vi "Periodic Tasks.vi"(8 "error in":errorcluster) -> ()   [LabVIEW 2015]
doc: "This VI runs in parallel to other tasks. It can contain as many user-defined periodic loops as you need. These can carry out PID or other sorts of timed response."
uses:
  <vilib>/Rock Robotics/WPI/Solenoid/WPI_SolenoidValue.ctl
  Robot Global Data.vi
  <vilib>/Rock Robotics/Network Tables/NT Write Boolean.vi
  <vilib>/Rock Robotics/WPI/Solenoid/WPI_SolenoidSetEnum.vi
  <vilib>/Rock Robotics/WPI/Utilities/WPI_GetSetVariantRefNum.vi
  <vilib>/Rock Robotics/WPI/RobotDrive/WPI_RobotDriveArcadeDrive_Standard(NoSaturation).vi
  <vilib>/Rock Robotics/Network Tables/NT Read Number.vi
  <vilib>/Rock Robotics/Network Tables/NT Read Numeric Array.vi
  <vilib>/Rock Robotics/Network Tables/NT Read Boolean.vi
  <vilib>/Rock Robotics/Network Tables/NT Write Number.vi
  navX Library v2/navX Library v2.lvlib
panel:
  in  "memoryStartAsSlow":dbl=0.3
  in  "min thresh 5":dbl=5e-05 format="%#_13g"
  in  "add if slow 5":dbl=0.007 format="%#_13g"
  in  "add if fast 5":dbl format="%#_13g"
  in  "turnSpeedStartSlow":dbl=0.3
  in  "distToStartAsSlow":dbl=0.2 format="%#_13g"
  in  "turnSpeedHard":dbl=0.5 format="%#_13g"
  in  "maxhi 2":dbl=0.8
  in  "high max 2":dbl=1.0
  in  "maxhi":dbl=0.65
  in  "turnSpeedSlow":dbl=0.37 format="%#_13g"
  in  "add if fast 4":dbl format="%#_13g"
  in  "add if slow 4":dbl=0.01 format="%#_13g"
  in  "min thresh 4":dbl=5e-05 format="%#_13g"
  out "aimState":i32
  in  "holding":dbl=0.25 format="%#_13g"
  in  "turnSpeed 7":dbl=0.37 format="%#_13g"
  in  "turnSpeedMedium":dbl=0.45 format="%#_13g"
  out "Target Angle 3":dbl=-17.534194944028258 format="%#_13g"
  in  "Angle 2":dbl=5.0 format="%#_13g"
  in  "cameraTarget 3":dbl=-0.03 format="%#_13g"
  in  "viewAngle 3":dbl=37.0 format="%#_13g"
  in  "arm vert offset":dbl=0.24 format="%#_13g"
  in  "arm horiz offset":dbl=0.07 format="%#_13g"
  out "leftOrRight":dbl=1.0
  in  "aimTolerance 2":dbl=6.0
  in  "high max":dbl=1.0
  in  "tapeRuntime":i32=25
  out "timeSaved 3":i32=27312
  in  "shiftthesh":dbl=0.67 format="%#_13g"
  in  "practiceOffset":dbl=-0.025 format="%#_13g"
  in  "tapeInPTO":dbl=-0.7
  out "timeSaved 2":i32=27123
  in  "left wait time":u32=13
  out "timeSaved":i32=14839
  in  "right wait time":u32=7
  out "LeftPin":bool
  out "RightPin":bool=TRUE
  in  "tapeOut":dbl=1.0 format="%#_13g"
  in  "tapeIn":dbl=-0.5 format="%#_13g"
  in  "tapeReturnSpeed":dbl
  in  "PTO speed":dbl=-1.0 format="%#_13g"
  in  "forceLowGear":bool
  out "voltage (V) 3":dbl=12.15
  out "Retainer Locked On":bool
  in  "y-override speed":dbl=-0.6 format="%#_13g"
  in  "Y-overide":bool
  in  "aimBot":dbl
  in  "modifyArm":dbl
  in  "distToRaise":dbl=24.0 format="%#_13g"
  in  "distToLower":dbl format="%#_13g"
  out "arm pot":dbl=0.9054580314226414
  out "rememberEnc":dbl=43.89548625
  out "Yes":bool
  in  "arm cdf offset":dbl=0.12
  in  "intake hi":dbl=-0.8
  out "arm output":dbl=-0.0 format="%.2f"
  # "This is all related to the auto-aim"
  # "These are what happens when starting close to the goal"
  # "ARM STUFF"
  # "auto-CDF"
  # "affects drive train:"
  # "minor high gear restrictions"
  # "Everything related to tape measures"
  # "9 and 16"
  # "practice 11 and 19"
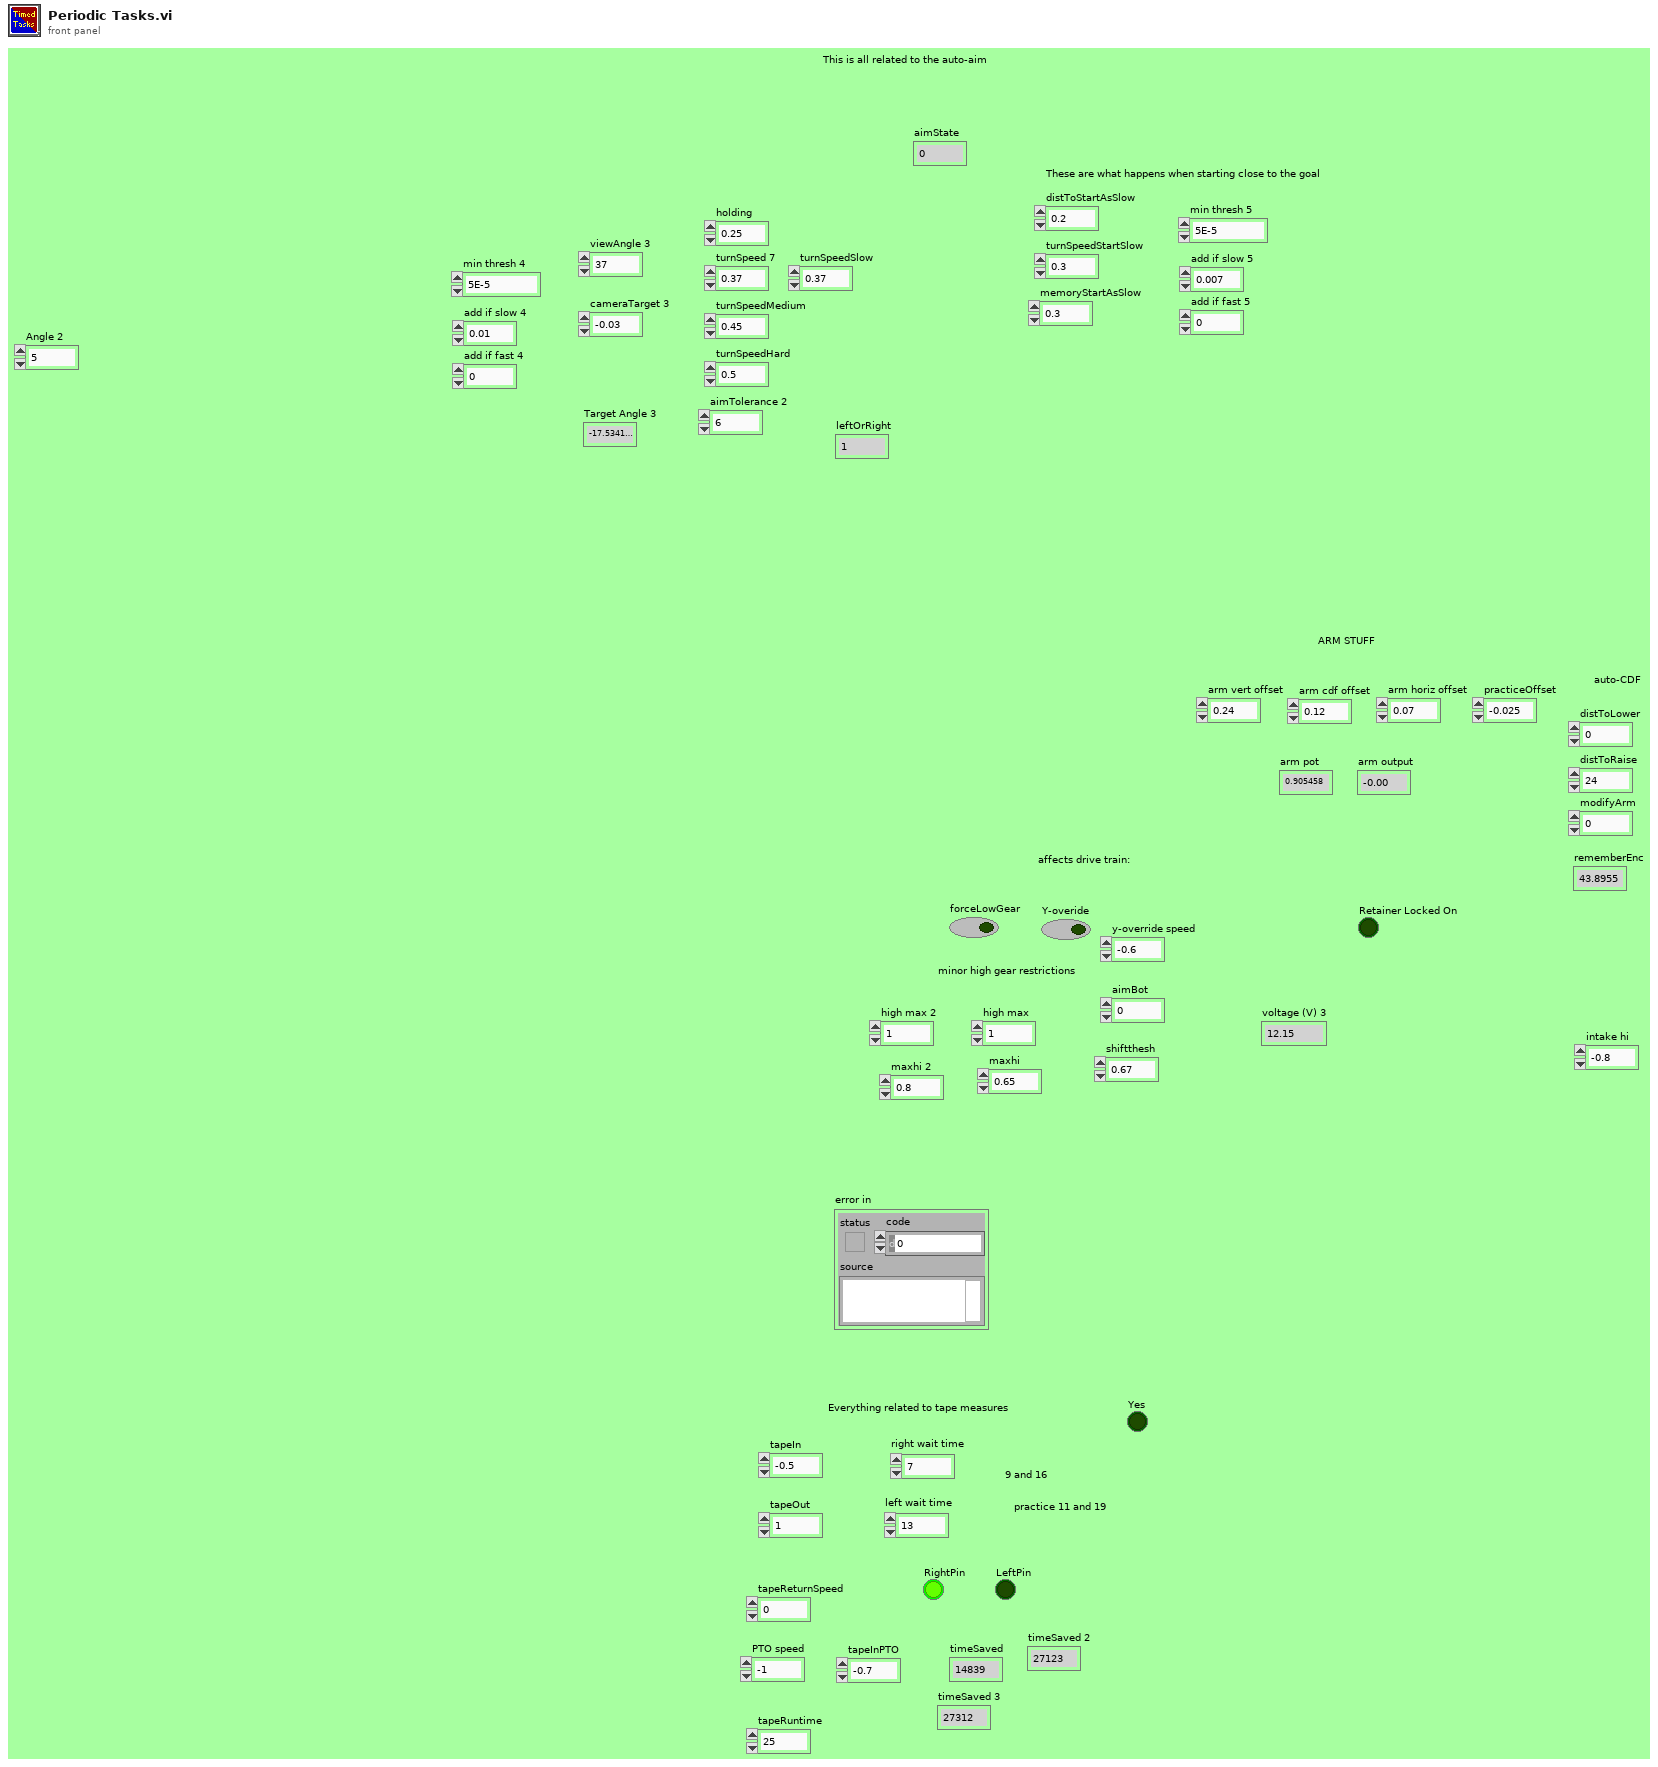
[diagram p1: front panel]
types:
  T1 = typedef "WPI_SolenoidDevRef.ctl" = cluster{"DevStatus":errorcluster, "Pneumatics Control Module":u8, "Forward Solenoid Channel":T2, "Reverse Solenoid Channel":T2}
  T2 = typedef "WPI_SolenoidChannel.ctl" = enum8{"Solenoid 0", "Solenoid 1", "Solenoid 2", "Solenoid 3", "Solenoid 4", "Solenoid 5", "Solenoid 6", "Solenoid 7", "Invalid"}
  T3 = typedef "WPI_RobotDriveDevRef.ctl" = cluster{"DevStatus":errorcluster, "Motors[]":T4[], "Square Inputs":bool, "Max Output":dbl}
  T4 = typedef "WPI_MotorControlDeviceRef.ctl" = cluster{"DeviceStatus":errorcluster, "Type":T5, "PWM":cluster{"PWM Channel":T6, "DeadBand":T7}, "CAN":cluster{"Device Number":u8, "Control Mode":T8, "Semaphore":T9, "Max Vout":dbl, "TalonSRX Control Mode":T10}, "Invert":bool}
  T5 = typedef "WPI_MotorControlType.ctl" = enum16{"PWM", "CAN", "CANTalonSRX"}
  T6 = typedef "FPGA_DIOPWMChannel.ctl" = enum8{"PWM 0", "PWM 1", "PWM 2", "PWM 3", "PWM 4", "PWM 5", "PWM 6", "PWM 7", "PWM 8", "PWM 9", "PWM MXP 0", "PWM MXP 1", "PWM MXP 2", "PWM MXP 3", "PWM MXP 4", "PWM MXP 5", "PWM MXP 6", "PWM MXP 7", "PWM MXP 8", "PWM MXP 9", "Invalid"}
  T7 = typedef "WPI_PWMDeadband.ctl" = cluster{"Name":string, "maxPositivePwm":i32, "minPositivePwm":i32, "centerPwm":i32, "maxNegativePwm":i32, "minNegativePwm":i32, "angularRange":u16}
  T8 = typedef "WPI_CANJaguar_ControlMode.ctl" = enum8{"Percent VBus", "Current", "Speed", "Position", "Voltage"}
  T9 = typedef "Semaphore RefNum" = refnum<k1>
  T10 = typedef "WPI_CANTalonSRX_APIControlMode.ctl" = enum8{"Percent VBus", "Speed", "Position", "Slave", "Unchanged / Invalid", "Voltage Compensation", "Current", "Motion Profile"}
  T11 = typedef "WPI_EncoderDevRef.ctl" = cluster{"DevStatus":errorcluster, "EncoderIndex":T12, "CounterIndex":T13, "DistancePerCount":dbl, "Decoding Type":T14}
  T12 = typedef "FPGA_EncoderIdx.ctl" = enum8{"Enc 0", "Enc 1", "Enc 2", "Enc 3", "Enc 4", "Enc 5", "Enc 6", "Enc 7", "Invalid"}
  T13 = typedef "FPGA_CounterCtrSystemIndex.ctl" = enum8{"Ctr 0", "Ctr 1", "Ctr 2", "Ctr 3", "Ctr 4", "Ctr 5", "Ctr 6", "Ctr 7", "Invalid"}
  T14 = typedef "WPI_EncoderType.ctl" = enum16{"1x", "2x", "4x"}
  T15 = typedef "WPI_DigitalInputDevRef.ctl" = cluster{"DevStatus":errorcluster, "DIO Channel":T16}
  T16 = typedef "FPGA_DIOChannel.ctl" = enum8{"DIO 0", "DIO 1", "DIO 2", "DIO 3", "DIO 4", "DIO 5", "DIO 6", "DIO 7", "DIO 8", "DIO 9", "DIO MXP 0", "DIO MXP 1", "DIO MXP 2", "DIO MXP 3", "DIO MXP 4", "DIO MXP 5", "DIO MXP 6", "DIO MXP 7", "DIO MXP 8", "DIO MXP 9", "DIO MXP 10", "DIO MXP 11", "DIO MXP 12", "DIO MXP 13", "DIO MXP 14", "DIO MXP 15", "Invalid"}
  T17 = typedef "WPI_PotentiometerDevRef.ctl" = cluster{"DevStatus":errorcluster, "Analog Channel":T18, "Invert Output":bool}
  T18 = typedef "FPGA_AIChannel.ctl" = enum8{"AI 0", "AI 1", "AI 2", "AI 3", "AI MXP 0", "AI MXP 1", "AI MXP 2", "AI MXP 3", "Invalid"}
  T19 = typedef "WPI_AnalogChannelDevRef.ctl" = cluster{"DevStatus":errorcluster, "Analog Channel":T18}
  T20 = typedef "navX Library v2.lvlib/Z900_navX_DeviceTypeDef.ctl" = cluster{"Interface":cluster{"Protocol":T21, "Update Rate (4Hz-60Hz)":u8, "navX Open TypeDef":variant}, "Notify Packet":refnum<notifier>, "Loop VI Refnum":refnum<vi>, "Ready to Close Occurrence Refnum":refnum<k4>}
  T21 = typedef "navX Library v2.lvlib/Z900_navX_ProtocolTypeDef.ctl" = enum16{"SERIAL", "I2C", "SPI"}
  T22 = typedef "WPI_CompressorDevRef.ctl" = cluster{"DevStatus":errorcluster, "Pneumatics Control Module":u8}
  T23 = cluster{"Yaw":dbl, "Roll":dbl, "Pitch":dbl, "Heading":dbl, "Fused Heading":dbl}
  T24 = typedef "WPI_SolenoidValue.ctl" = enum16{"Off", "On", "Forward", "Reverse"}
  T25 = cluster{"SolenoidDevRef":T1, "SolenoidDevRef":T1, "SolenoidDevRef":T1, "SolenoidDevRef":T1}
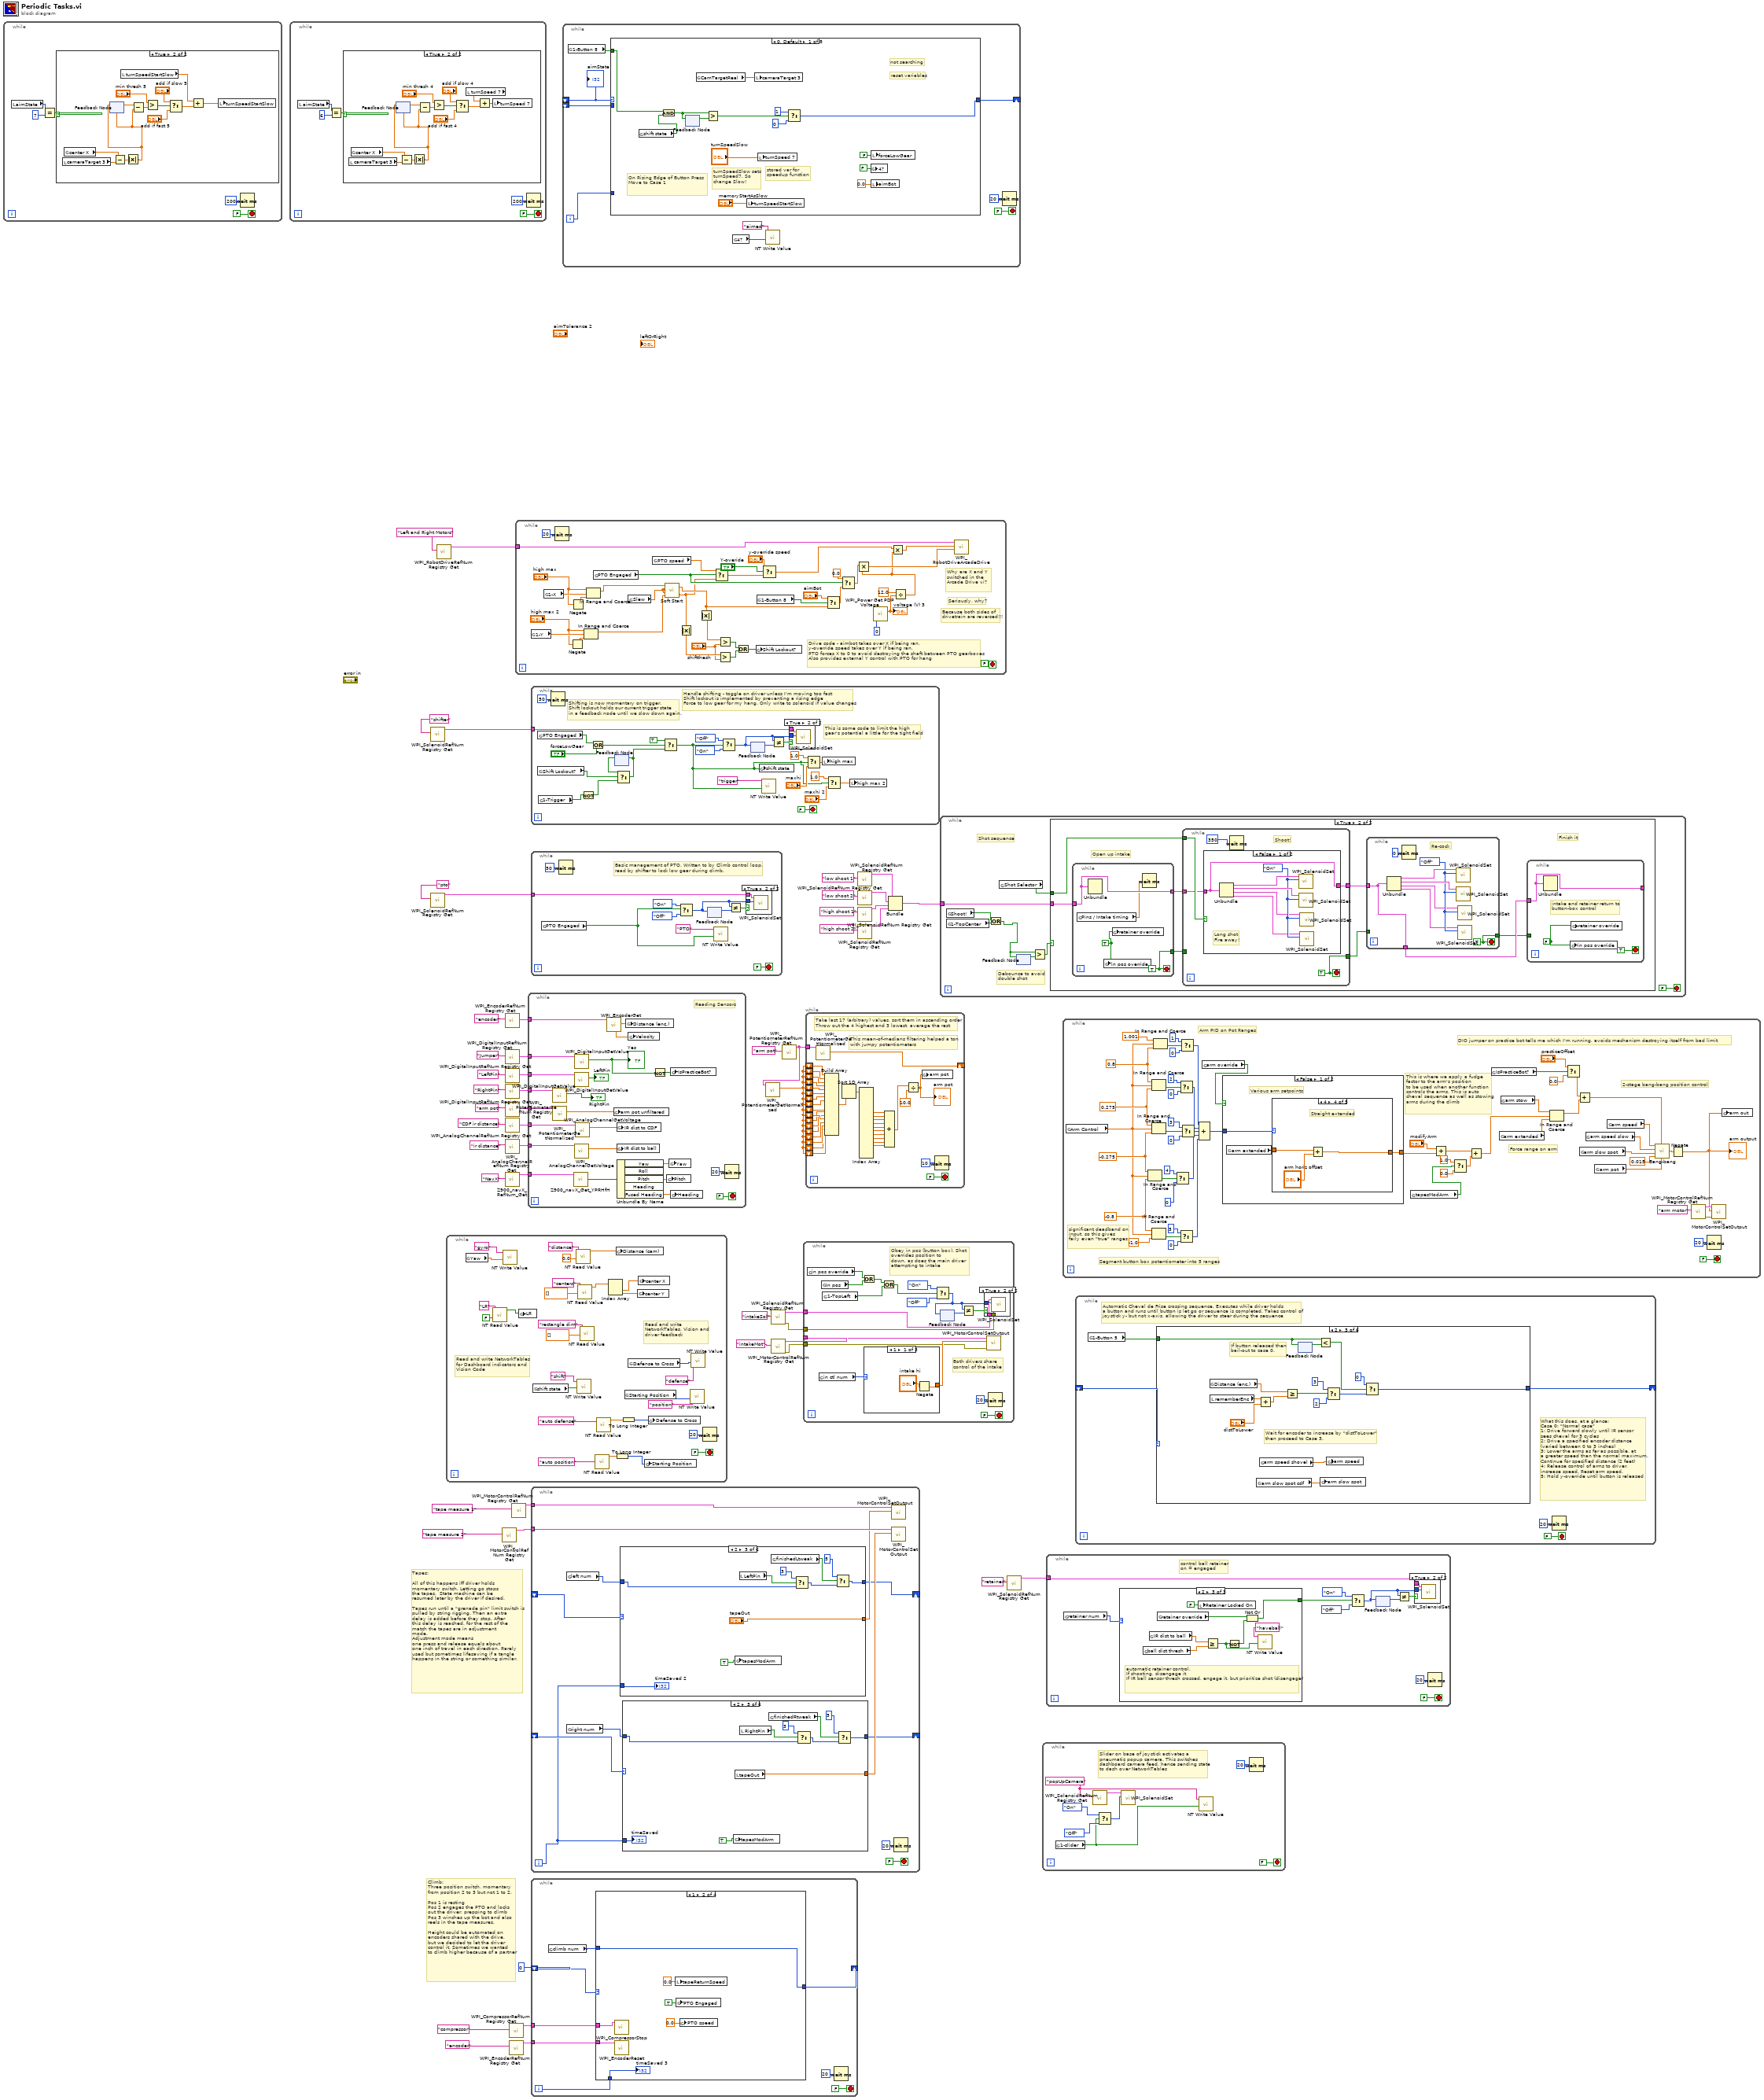
[diagram p0: block diagram]
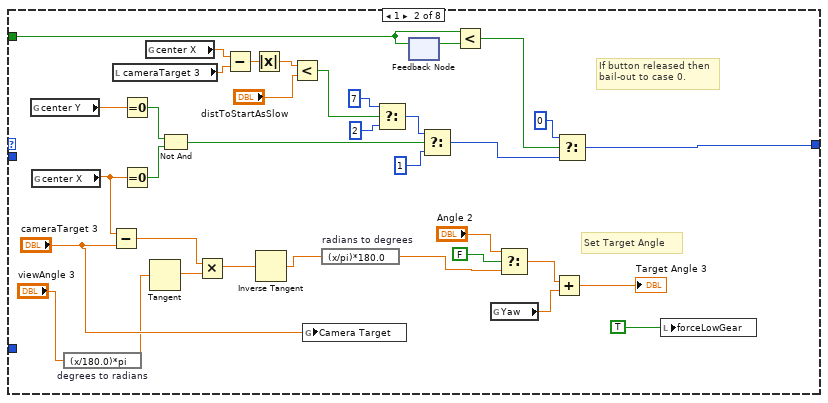
[diagram p4: hidden frame]
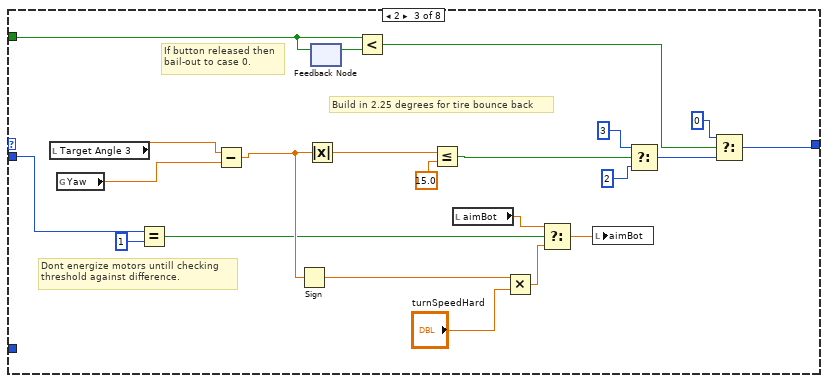
[diagram p5: hidden frame]
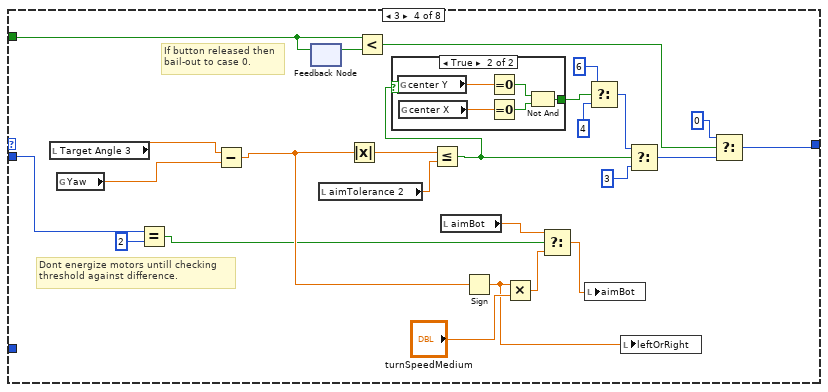
[diagram p6: hidden frame]
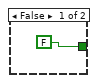
[diagram p7: hidden frame]
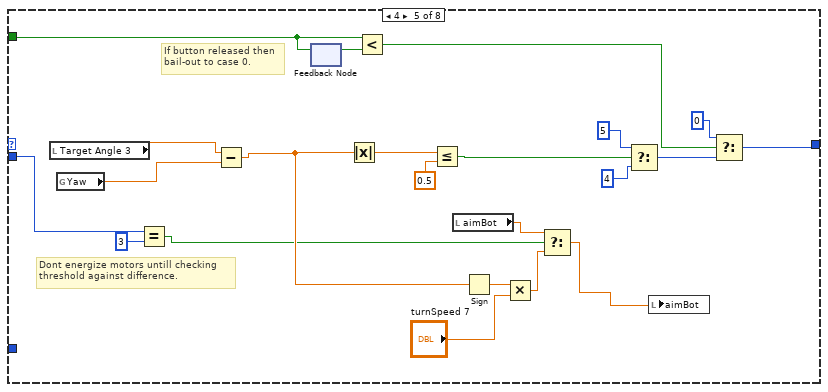
[diagram p8: hidden frame]
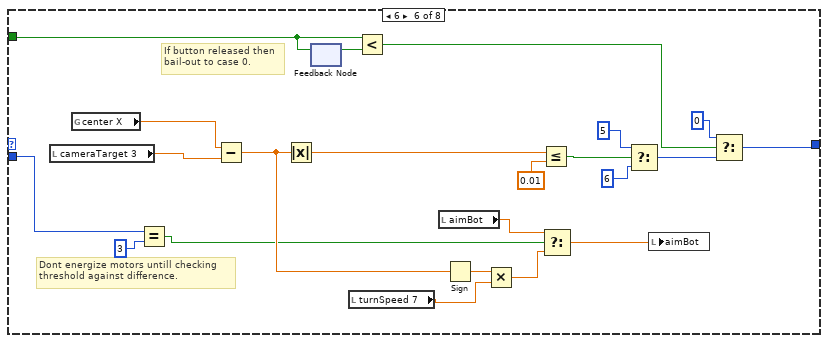
[diagram p9: hidden frame]
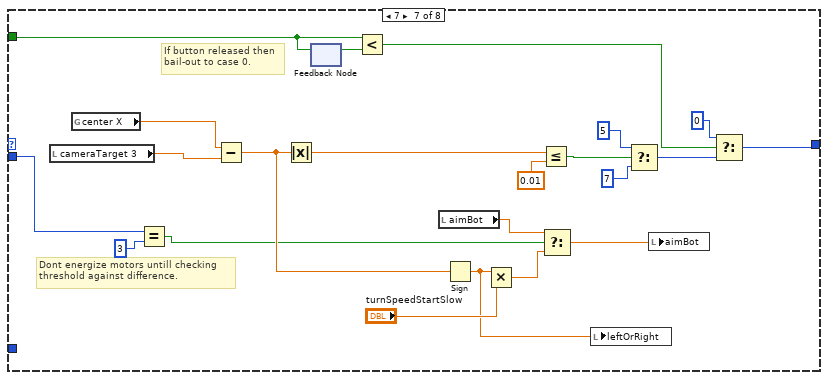
[diagram p10: hidden frame]
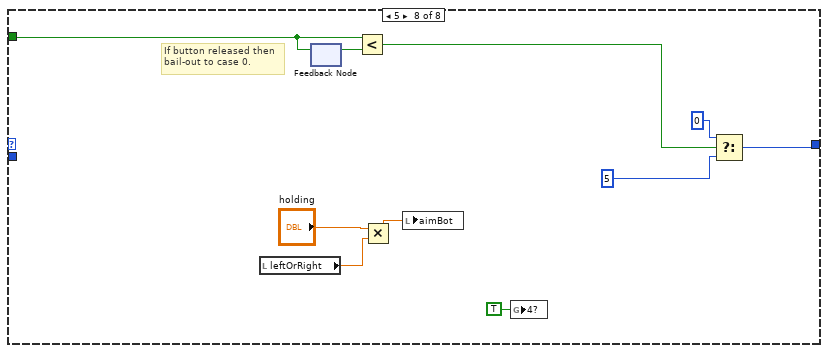
[diagram p11: hidden frame]
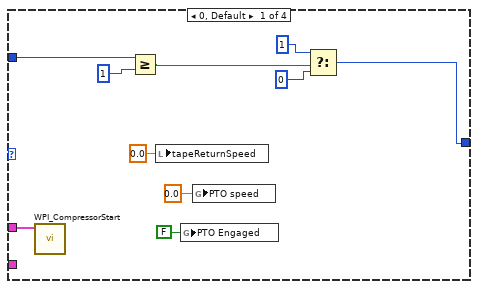
[diagram p12: hidden frame]
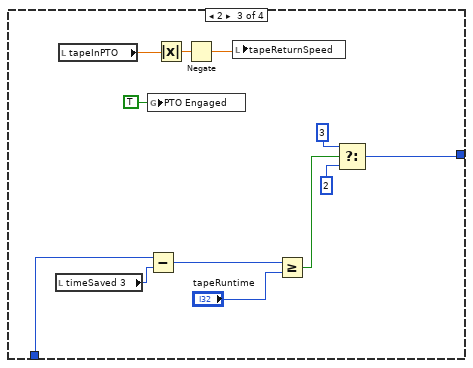
[diagram p13: hidden frame]
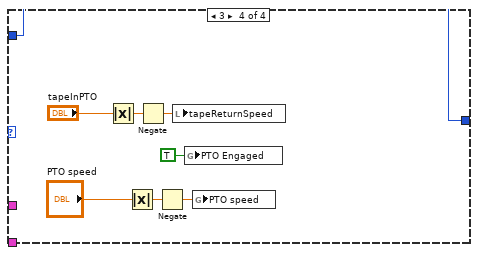
[diagram p14: hidden frame]
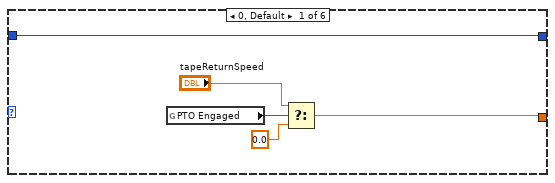
[diagram p15: hidden frame]
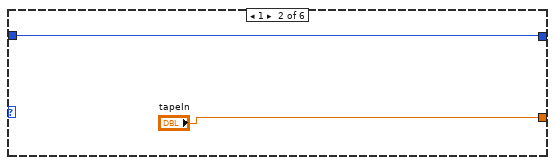
[diagram p16: hidden frame]
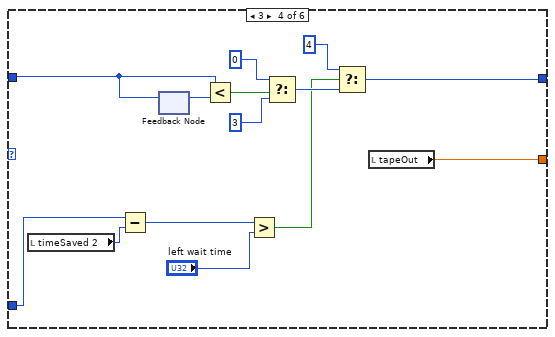
[diagram p17: hidden frame]
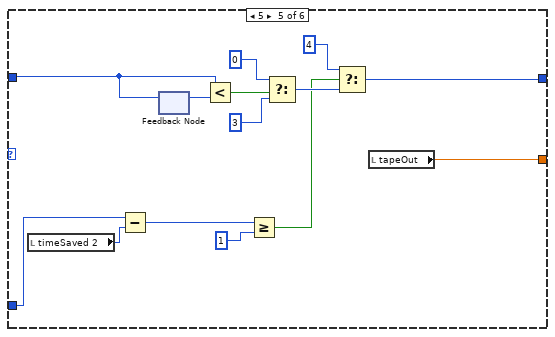
[diagram p18: hidden frame]
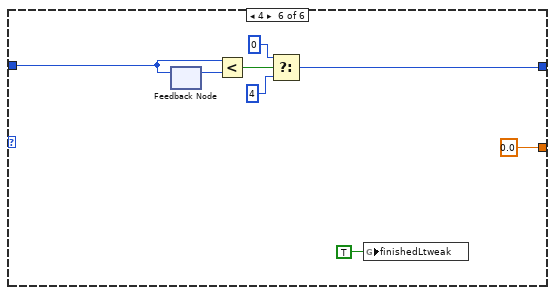
[diagram p19: hidden frame]
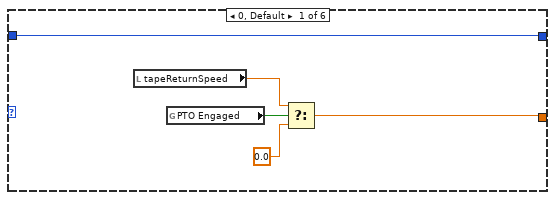
[diagram p20: hidden frame]
diagram:
  # "Climb:\nThree position switch, momentary\nfrom position 2 to 3 but not 1 to 2.\n\nPos 1 is resting\nPos 2 engages the PTO and locks\nout the driver, prepping to climb\nPos 3 winches up the bot and also\nreels in the tape measures.\n\nHeight could be automated on\nencoders shared with the drive,\nbut we decided to let the driver\ncontrol it. Sometimes we wanted\nto climb higher because of a partner"
  # "Tapes:\n\nAll of this happens iff driver holds\nmomentary switch. Letting go stops\nthe tapes.  State machine can be\nresumed later by the driver if desired.\n\nTapes run until a \"grenade pin\" limit switch is\npulled by string rigging. Then an extra\ndelay is added before they stop. After\nthis delay is reached, for the rest of the\nmatch the tapes are in adjustment\nmode. \nAdjustment mode means\none press and release equals about \none inch of travel in each direction. Rarely\nused but sometimes lifesaving if a tangle \nhappens in the string or something similar."
  n1 = while {
    stop <- FALSE stop-if-true
    n2 = local read "aimState"() -> (w54:i32)
    n3 = Equal?(x=w54, y=7) -> (x = y?=w52:bool)
    n4 = case shown="True" w52 {
      frame False {
      }
      frame True {
        n5 = local read "cameraTarget 3"() -> (w68:dbl)
        n6 = global read "Robot Global Data.vi" "center X"() -> (w69:dbl)
        n7 = Subtract(x=w69, y=w68) -> (x-y=w58:dbl)
        n8 = local read "turnSpeedStartSlow"() -> (w60:dbl)
        n9 = Absolute Value(x=w58) -> (abs(x)=w57:dbl)
        n10 = feedback #1(w57) -> (w66:dbl)
        n11 = feedback-in #1(w57) -> ()
        n12 = Subtract(x=w66, y=w57) -> (x-y=w65:dbl)
        n13 = Greater?(x="min thresh 5", y=w65) -> (0:w63:bool)
        n14 = Select(t="add if slow 5", s=w63, f="add if fast 5") -> (s? t:f=w61:dbl)
        n15 = Add(x=w60, y=w61) -> (x+y=w59:dbl)
        n16 = local write "turnSpeedStartSlow"(w59) -> ()
      }
    }
    n17 = Wait (ms)(milliseconds to wait=u32 200) -> ()  [unwired: 1 out]
  }
  n18 = while {
    stop <- FALSE stop-if-true
    n19 = local read "aimState"() -> (w72:i32)
    n20 = Equal?(x=w72, y=6) -> (x = y?=w70:bool)
    n21 = case shown="True" w70 {
      frame False {
      }
      frame True {
        n22 = local read "cameraTarget 3"() -> (w86:dbl)
        n23 = global read "Robot Global Data.vi" "center X"() -> (w87:dbl)
        n24 = Subtract(x=w87, y=w86) -> (x-y=w76:dbl)
        n25 = Absolute Value(x=w76) -> (abs(x)=w75:dbl)
        n26 = feedback #2(w75) -> (w84:dbl)
        n27 = feedback-in #2(w75) -> ()
        n28 = Subtract(x=w84, y=w75) -> (x-y=w83:dbl)
        n29 = Greater?(x="min thresh 4", y=w83) -> (0:w81:bool)
        n30 = Select(t="add if slow 4", s=w81, f="add if fast 4") -> (s? t:f=w79:dbl)
        n31 = local read "turnSpeed 7"() -> (w78:dbl)
        n32 = Add(x=w78, y=w79) -> (x+y=w77:dbl)
        n33 = local write "turnSpeed 7"(w77) -> ()
      }
    }
    n34 = Wait (ms)(milliseconds to wait=u32 200) -> ()  [unwired: 1 out]
  }
  n35 = call <vilib>:"WPI_SolenoidRefNum Registry Get.vi"("refnum name"="shifter") -> ("SolenoidDevRef"=w50:T1)  [unwired: 9 in, 1 out]
  n36 = call <vilib>:"WPI_SolenoidRefNum Registry Get.vi"("refnum name"="pto") -> ("SolenoidDevRef"=w46:T1)  [unwired: 9 in, 1 out]
  n37 = call <vilib>:"WPI_RobotDriveRefNum Registry Get.vi"("refnum name"="Left and Right Motors") -> ("RobotDriveDevRef"=w48:T3)  [unwired: 9 in, 1 out]
  n38 = while {
    stop <- FALSE stop-if-true
    # "Read and write NetworkTables\nfor Dashboard indicators and\nVision Code"
    # "Read and write NetworkTables. Vision and driver feedback"
    n39 = global read "Robot Global Data.vi" "Yaw"() -> (w91:dbl)
    n40 = call-poly <vilib>:"NT Read Value.vi"("Default Value"=FALSE, "Name"="LR") -> ("Boolean"=w88:bool)  [unwired: 8 in, 1 out]
    n41 = call-poly <vilib>:"NT Write Value.vi"("Numeric"=w91, "Name"="gyro") -> ()  [unwired: 9 in, 1 out]
    n42 = global write "Robot Global Data.vi" "LR"(w88) -> ()
    n43 = global read "Robot Global Data.vi" "shift state"() -> (w104:bool)
    n44 = call-poly <vilib>:"NT Read Value.vi"("Default Value"=0.0, "Name"="distance") -> ("Numeric"=w109:dbl)  [unwired: 8 in, 1 out]
    n45 = call-poly <vilib>:"NT Write Value.vi"("Boolean"=w104, "Name"="shift") -> ()  [unwired: 9 in, 1 out]
    n46 = call-poly <vilib>:"NT Read Value.vi"("Default Value"=dbl[] [], "Name"="centers") -> ("Numeric Array"=w108:dbl[])  [unwired: 8 in, 1 out]
    n47 = call-poly <vilib>:"NT Read Value.vi"("Default Value"=dbl[] [], "Name"="rectangle dim") -> ()  [unwired: 8 in, 2 out]
    n48 = call-poly <vilib>:"NT Read Value.vi"("Name"="auto position") -> ("Numeric"=w100:dbl)  [unwired: 9 in, 1 out]
    n49 = call-poly <vilib>:"NT Read Value.vi"("Name"="auto defense") -> ("Numeric"=w99:dbl)  [unwired: 9 in, 1 out]
    n50 = Index Array(array=w108) -> (element #1=w107:dbl, element #2=w106:dbl)  [unwired: 2 in]
    n51 = To Long Integer(number=w100) -> (32bit integer=w97:i32)
    n52 = global write "Robot Global Data.vi" "Distance (cam)"(w109) -> ()
    n53 = To Long Integer(number=w99) -> (32bit integer=w98:i32)
    n54 = global read "Robot Global Data.vi" "Starting Position"() -> (w95:i32)
    n55 = global read "Robot Global Data.vi" "Defense to Cross"() -> (w96:i32)
    n56 = global write "Robot Global Data.vi" "center Y"(w106) -> ()
    n57 = global write "Robot Global Data.vi" "center X"(w107) -> ()
    n58 = global write "Robot Global Data.vi" "Starting Position"(w97) -> ()
    n59 = global write "Robot Global Data.vi" "Defense to Cross"(w98) -> ()
    n60 = call-poly <vilib>:"NT Write Value.vi"("Numeric"=w95, "Name"="position") -> ()  [unwired: 9 in, 1 out]
    n61 = call-poly <vilib>:"NT Write Value.vi"("Numeric"=w96, "Name"="defense") -> ()  [unwired: 9 in, 1 out]
    n62 = Wait (ms)(milliseconds to wait=u32 20) -> ()  [unwired: 1 out]
  }
  n63 = call <vilib>:"WPI_MotorControlRefNum Registry Get.vi"("refnum name"="tape measure 2") -> ("MotorControlDevRef"=w25:T4)  [unwired: 9 in, 1 out]
  n64 = call <vilib>:"WPI_EncoderRefNum Registry Get.vi"("refnum name"="encoder") -> ("EncoderDevRef"=w8:T11)  [unwired: 9 in, 1 out]
  n65 = call <vilib>:"WPI_DigitalInputRefNum Registry Get.vi"("refnum name"="Jumper") -> ("DigitalInputDevRef"=w7:T15)  [unwired: 9 in, 1 out]
  n66 = call <vilib>:"WPI_DigitalInputRefNum Registry Get.vi"("refnum name"="LeftPin") -> ("DigitalInputDevRef"=w6:T15)  [unwired: 9 in, 1 out]
  n67 = call <vilib>:"WPI_DigitalInputRefNum Registry Get.vi"("refnum name"="RightPin") -> ("DigitalInputDevRef"=w5:T15)  [unwired: 9 in, 1 out]
  n68 = call <vilib>:"WPI_PotentiometerRefNum Registry Get.vi"("refnum name"="arm pot") -> ("PotDevRef"=w4:T17)  [unwired: 9 in, 1 out]
  n69 = call <vilib>:"WPI_AnalogChannelRefNum Registry Get.vi"("refnum name"="CDF ir distance") -> ("AIDeviceRef"=w3:T19)  [unwired: 9 in, 1 out]
  n70 = call <vilib>:"WPI_AnalogChannelRefNum Registry Get.vi"("refnum name"="ir distance") -> ("AIDeviceRef"=w2:T19)  [unwired: 9 in, 1 out]
  n71 = call "Z900_navX_RefNum_Get.vi"("refnum name"="NavX") -> ("navX Device"=w1:T20)  [unwired: 9 in, 1 out]
  n72 = call <vilib>:"WPI_CompressorRefNum Registry Get.vi"("refnum name"="compressor") -> ("CompressorDevRef"=w21:T22)  [unwired: 9 in, 1 out]
  n73 = call <vilib>:"WPI_EncoderRefNum Registry Get.vi"("refnum name"="encoder") -> ("EncoderDevRef"=w23:T11)  [unwired: 9 in, 1 out]
  n74 = call <vilib>:"WPI_MotorControlRefNum Registry Get.vi"("refnum name"="tape measure 1") -> ("MotorControlDevRef"=w28:T4)  [unwired: 9 in, 1 out]
  n75 = while {
    tunnel: w48 -> [w151]
    stop <- FALSE stop-if-true
    # "Because both sides of \ndrivetrain are reversed!!!"
    # "Drive code - aimbot takes over X if being ran,\ny-override speed takes over Y if being ran, \nPTO forces X to 0 to avoid destroying the shaft between PTO gearboxes\nAlso provides external Y control with PTO for hang"
    # "Seriously, why?"
    # "Why are X and Y switched in the Arcade Drive vi?"
    n76 = global read "Robot Global Data.vi" "1-Y"() -> (w124:dbl)
    n77 = global read "Robot Global Data.vi" "1-X"() -> (w125:dbl)
    n78 = Wait (ms)(milliseconds to wait=u32 20) -> ()  [unwired: 1 out]
    n79 = Negate(x="high max 2") -> (-x=w122:dbl)
    n80 = Negate(x="high max") -> (-x=w123:dbl)
    n81 = In Range and Coerce(upper limit="high max 2", x=w124, lower limit=w122) -> (coerced(x)=w119:dbl)  [unwired: 1 out]
    n82 = In Range and Coerce(upper limit="high max", x=w125, lower limit=w123) -> (coerced(x)=w120:dbl)  [unwired: 1 out]
    n83 = global read "Robot Global Data.vi" "PTO Engaged"() -> (w146:bool)
    n84 = global read "Robot Global Data.vi" "Slew"() -> (w117:dbl)
    n85 = global read "Robot Global Data.vi" "PTO speed"() -> (w147:dbl)
    n86 = call "Soft Start.vi"("Y-axis Joystick"=w119, "Y-Slew Rate"=w117, "X-Slew Rate"=w117, "X- axis Joystick"=w120) -> ("Y-axis drive"=w126:dbl, "X-axis drive"=w127:dbl)
    n87 = Absolute Value(x=w126) -> (abs(x)=w144:dbl)
    n88 = Absolute Value(x=w127) -> (abs(x)=w145:dbl)
    n89 = Select(t=w147, s=w146, f=w126) -> (s? t:f=w139:dbl)
    n90 = Greater?(x=w144, y="shiftthesh") -> (0:w150:bool)
    n91 = Greater?(x=w145, y="shiftthesh") -> (0:w148:bool)
    n92 = Or(x=w148, y=w150) -> (x .or. y?=w149:bool)
    n93 = global write "Robot Global Data.vi" "Shift Lockout?"(w149) -> ()
    n94 = global read "Robot Global Data.vi" "1-Button 8"() -> (w140:bool)
    n95 = Select(t="y-override speed", s="Y-overide", f=w139) -> (s? t:f=w131:dbl)
    n96 = Select(t="aimBot", s=w140, f=w127) -> (s? t:f=w141:dbl)
    n97 = Select(t=0.0, s=w146, f=w141) -> (s? t:f=w133:dbl)
    n98 = call <vilib>:"WPI_Power Get PDP Voltage.vi"("Power Distribution Panel (0)"=u8 0) -> ("voltage (V)"=w135:dbl)  [unwired: 13 in, 1 out]
    "voltage (V) 3" <- w135
    n99 = Divide(x=12.0, y=w135) -> (x/y=w130:dbl)
    n100 = Multiply(x=w133, y=w130) -> (x*y=w132:dbl)
    n101 = Multiply(x=w131, y=w130) -> (x*y=w129:dbl)
    n102 = call-poly <vilib>:"WPI_RobotDriveArcadeDrive.vi"("Y axis value"=w132, "X axis value"=w129, "RobotDriveDevRef"=w151) -> ()  [unwired: 6 in, 3 out]
  }
  n103 = while {
    tunnel: w8 -> [w161]
    tunnel: w7 -> [w160]
    tunnel: w6 -> [w159]
    tunnel: w5 -> [w158]
    tunnel: w4 -> [w157]
    tunnel: w3 -> [w156]
    tunnel: w2 -> [w155]
    tunnel: w1 -> [w154]
    stop <- FALSE stop-if-true
    # "Reading Sensors"
    n104 = call <vilib>:"WPI_DigitalInputGetValue.vi"("DigitalInputDevRef"=w158) -> ("Value"=→"RightPin":bool)  [unwired: 8 in, 2 out]
    n105 = call <vilib>:"WPI_PotentiometerGetNormalized.vi"("PotDevRef"=w157) -> ("Normalized Value"=w168:dbl)  [unwired: 8 in, 2 out]
    n106 = call "Z900_navX_Get_YPRHfH.vi"("navX Device"=w154) -> ("YRPHfH"=w167:T23)  [unwired: 7 in, 3 out]
    n107 = call <vilib>:"WPI_DigitalInputGetValue.vi"("DigitalInputDevRef"=w159) -> ("Value"=→"LeftPin":bool)  [unwired: 8 in, 2 out]
    n108 = call <vilib>:"WPI_AnalogChannelGetVoltage.vi"("AIDeviceRef"=w155) -> ("Voltage"=w170:dbl)  [unwired: 8 in, 2 out]
    n109 = call <vilib>:"WPI_DigitalInputGetValue.vi"("DigitalInputDevRef"=w160) -> ("Value"=w172:bool)  [unwired: 8 in, 2 out]
    "Yes" <- w172
    n110 = call <vilib>:"WPI_AnalogChannelGetVoltage.vi"("AIDeviceRef"=w156) -> ("Voltage"=w169:dbl)  [unwired: 8 in, 2 out]
    n111 = call <vilib>:"WPI_EncoderGet.vi"("EncoderDevRef"=w161) -> ("Distance"=w174:dbl, "Rate"=w173:dbl)  [unwired: 5 in, 4 out]
    n112 = global write "Robot Global Data.vi" "arm pot unfiltered"(w168) -> ()
    n113 = global write "Robot Global Data.vi" "IR dist to CDF"(w169) -> ()
    n114 = global write "Robot Global Data.vi" "IR dist to ball"(w170) -> ()
    n115 = Unbundle By Name(w167) -> ("Yaw"=w166:dbl, "Pitch"=w165:dbl, "Fused Heading"=w164:dbl)  [unwired: 2 out]
    n116 = global write "Robot Global Data.vi" "Distance (enc.)"(w174) -> ()
    n117 = global write "Robot Global Data.vi" "Velocity"(w173) -> ()
    n118 = Not(x=w172) -> (.not. x?=w171:bool)
    n119 = global write "Robot Global Data.vi" "Pitch"(w165) -> ()
    n120 = global write "Robot Global Data.vi" "Yaw"(w166) -> ()
    n121 = global write "Robot Global Data.vi" "IsPracticeBot?"(w171) -> ()
    n122 = global write "Robot Global Data.vi" "Heading"(w164) -> ()
    n123 = Wait (ms)(milliseconds to wait=u32 20) -> ()  [unwired: 1 out]
  }
  n124 = while {
    tunnel: w50 -> [w194]
    stop <- FALSE stop-if-true
    # "This is some code to limit the high\ngear's potential a little for the tight field"
    # "Shifting is now momentary on trigger.\nShift lockout holds our current trigger state\nin a feedback node until we slow down again."
    # "Handle shifting - toggle on driver unless I'm moving too fast\nShift lockout is implemented by preventing a rising edge\nForce to low gear for my hang. Only write to solenoid if value changes"
    n125 = global read "Robot Global Data.vi" "PTO Engaged"() -> (w188:bool)
    n126 = global read "Robot Global Data.vi" "Shift Lockout?"() -> (w190:bool)
    n127 = global read "Robot Global Data.vi" "1-Trigger"() -> (w185:bool)
    n128 = Wait (ms)(milliseconds to wait=u32 50) -> ()  [unwired: 1 out]
    n129 = Not(x=w185) -> (.not. x?=w184:bool)
    n130 = Or(x=w188, y="forceLowGear") -> (x .or. y?=w187:bool)
    n131 = feedback #3() -> (w191:bool)  [unwired: 1 in]
    n132 = Select(t=w191, s=w190, f=w184) -> (s? t:f=w189:bool)
    n133 = feedback-in #3(w189) -> ()
    n134 = Select(t=TRUE, s=w187, f=w189) -> (s? t:f=w177:bool)
    n135 = Select(t=WPI_SolenoidValue."Off" ("Value"), s=w177, f=WPI_SolenoidValue."On" ("Value")) -> (s? t:f=w192:T24)
    n136 = feedback #4() -> (w195:T24)  [unwired: 1 in]
    n137 = feedback-in #4(w192) -> ()
    n138 = global write "Robot Global Data.vi" "shift state"(w177) -> ()
    n139 = call-poly <vilib>:"NT Write Value.vi"("Boolean"=w177, "Name"="trigger") -> ()  [unwired: 9 in, 1 out]
    n140 = Not Equal?(x=w192, y=w195) -> (x != y?=w196:bool)
    n141 = case shown="True" w196 {
      tunnel: w192 -> [_ w203]
      tunnel: w194 -> [_ w202]
      frame False {
      }
      frame True {
        n142 = call-poly <vilib>:"WPI_SolenoidSet.vi"("Value"=w203, "SolenoidDevRef"=w202) -> ()  [unwired: 8 in, 2 out]
      }
    }
    n143 = Select(t=1.0, s=w177, f="maxhi") -> (s? t:f=w181:dbl)
    n144 = local write "high max"(w181) -> ()
    n145 = Select(t=1.0, s=w177, f="maxhi 2") -> (s? t:f=w179:dbl)
    n146 = local write "high max 2"(w179) -> ()
  }
  n147 = while {
    tunnel: w46 -> [w205]
    stop <- FALSE stop-if-true
    # "Basic management of PTO. Written to by Climb control loop,\nread by shifter to lock low gear during climb."
    n148 = global read "Robot Global Data.vi" "PTO Engaged"() -> (w204:bool)
    n149 = Wait (ms)(milliseconds to wait=u32 50) -> ()  [unwired: 1 out]
    n150 = Select(t=WPI_SolenoidValue."On" ("Value"), s=w204, f=WPI_SolenoidValue."Off" ("Value")) -> (s? t:f=w206:T24)
    n151 = feedback #5() -> (w207:T24)  [unwired: 1 in]
    n152 = feedback-in #5(w206) -> ()
    n153 = call-poly <vilib>:"NT Write Value.vi"("Boolean"=w204, "Name"="PTO") -> ()  [unwired: 9 in, 1 out]
    n154 = Not Equal?(x=w206, y=w207) -> (x != y?=w208:bool)
    n155 = case shown="True" w208 {
      tunnel: w206 -> [_ w215]
      tunnel: w205 -> [_ w214]
      frame False {
      }
      frame True {
        n156 = call-poly <vilib>:"WPI_SolenoidSet.vi"("Value"=w215, "SolenoidDevRef"=w214) -> ()  [unwired: 8 in, 2 out]
      }
    }
  }
  n157 = while {
    tunnel: w28 -> [w227]
    tunnel: w25 -> [w226]
    shift-right: [w222] -> _
    shift-left: _ -> [w223]
    shift-right: [w217] -> _
    shift-left: _ -> [w216]
    i -> [w219]
    stop <- FALSE stop-if-true
    n158 = global read "Robot Global Data.vi" "left num"() -> (w220:i8)
    n159 = global read "Robot Global Data.vi" "right num"() -> (w221:i8)
    n160 = case shown="2" w216 {
      tunnel: [w232 "tapeIn" "tapeOut" w252 w267 0.0] -> w218
      tunnel: w220 -> [w231 w235 w245 w256 w271 w280]
      tunnel: [w231 w235 w239 w247 w262 w276] -> w217
      tunnel: w219 -> [_ _ w241 w253 w268 _]
      frame 0, Default {
        n161 = global read "Robot Global Data.vi" "PTO Engaged"() -> (w233:bool)
        n162 = Select(t="tapeReturnSpeed", s=w233, f=0.0) -> (s? t:f=w232:dbl)
      }
      frame 1 {
      }
      frame 2 {
        n163 = global write "Robot Global Data.vi" "tapesModArm"(TRUE ("tapesModArm?")) -> ()
        n164 = local read "LeftPin"() -> (w243:bool)
        n165 = global read "Robot Global Data.vi" "finishedLtweak"() -> (w237:bool)
        n166 = Select(t=i8 3, s=w243, f=w245) -> (s? t:f=w238:i8)
        n167 = Select(t=i8 5, s=w237, f=w238) -> (s? t:f=w239:i8)
        "timeSaved 2" <- w241
      }
      frame 3 {
        n168 = local read "timeSaved 2"() -> (w246:i32)
        n169 = Subtract(x=w253, y=w246) -> (x-y=w259:i32)
        n170 = feedback #6() -> (w257:i8)  [unwired: 1 in]
        n171 = feedback-in #6(w256) -> ()
        n172 = Less?(x=w256, y=w257) -> (x < y?=w251:bool)
        n173 = Greater?(x=w259, y="left wait time") -> (0:w249:bool)
        n174 = Select(t=0, s=w251, f=3) -> (s? t:f=w250:i32)
        n175 = Select(t=4, s=w249, f=w250) -> (s? t:f=w247:i32)
        n176 = local read "tapeOut"() -> (w252:dbl)
      }
      frame 5 {
        n177 = local read "timeSaved 2"() -> (w261:i32)
        n178 = Subtract(x=w268, y=w261) -> (x-y=w273:i32)
        n179 = feedback #7() -> (w272:i8)  [unwired: 1 in]
        n180 = feedback-in #7(w271) -> ()
        n181 = Less?(x=w271, y=w272) -> (x < y?=w266:bool)
        n182 = Greater Or Equal?(x=w273, y=1) -> (x >= y?=w264:bool)
        n183 = Select(t=0, s=w266, f=3) -> (s? t:f=w265:i32)
        n184 = Select(t=4, s=w264, f=w265) -> (s? t:f=w262:i32)
        n185 = local read "tapeOut"() -> (w267:dbl)
      }
      frame 4 {
        n186 = feedback #8() -> (w281:i8)  [unwired: 1 in]
        n187 = feedback-in #8(w280) -> ()
        n188 = Less?(x=w280, y=w281) -> (x < y?=w279:bool)
        n189 = Select(t=0, s=w279, f=4) -> (s? t:f=w276:i32)
        n190 = global write "Robot Global Data.vi" "finishedLtweak"(TRUE ("finishedLtweak")) -> ()
      }
    }
    n191 = case shown="2" w223 {
      tunnel: [w285 w288 w298 w304 w319 0.0] -> w225
      tunnel: w221 -> [w284 w287 w297 w309 w324 w333]
      tunnel: [w284 w287 w291 w299 w314 w329] -> w222
      tunnel: w219 -> [_ _ w294 w306 w321 _]
      frame 0, Default {
        n192 = local read "tapeReturnSpeed"() -> (w283:dbl)
        n193 = global read "Robot Global Data.vi" "PTO Engaged"() -> (w286:bool)
        n194 = Select(t=w283, s=w286, f=0.0) -> (s? t:f=w285:dbl)
      }
      frame 1 {
        n195 = local read "tapeIn"() -> (w288:dbl)
      }
      frame 2 {
        n196 = global write "Robot Global Data.vi" "tapesModArm"(TRUE ("tapesModArm?")) -> ()
        n197 = local read "tapeOut"() -> (w298:dbl)
        n198 = local read "RightPin"() -> (w295:bool)
        n199 = global read "Robot Global Data.vi" "finishedRtweak"() -> (w290:bool)
        n200 = Select(t=i8 3, s=w295, f=w297) -> (s? t:f=w292:i8)
        n201 = Select(t=i8 5, s=w290, f=w292) -> (s? t:f=w291:i8)
        "timeSaved" <- w294
      }
      frame 3 {
        n202 = local read "timeSaved"() -> (w305:i32)
        n203 = Subtract(x=w306, y=w305) -> (x-y=w312:i32)
        n204 = feedback #9() -> (w310:i8)  [unwired: 1 in]
        n205 = feedback-in #9(w309) -> ()
        n206 = Less?(x=w309, y=w310) -> (x < y?=w303:bool)
        n207 = Greater?(x=w312, y="right wait time") -> (0:w301:bool)
        n208 = Select(t=0, s=w303, f=3) -> (s? t:f=w302:i32)
        n209 = Select(t=4, s=w301, f=w302) -> (s? t:f=w299:i32)
        n210 = local read "tapeOut"() -> (w304:dbl)
      }
      frame 5 {
        # "Manual Adjust Mode"
        n211 = local read "timeSaved"() -> (w320:i32)
        n212 = Subtract(x=w321, y=w320) -> (x-y=w326:i32)
        n213 = feedback #10() -> (w325:i8)  [unwired: 1 in]
        n214 = feedback-in #10(w324) -> ()
        n215 = Less?(x=w324, y=w325) -> (x < y?=w318:bool)
        n216 = Greater Or Equal?(x=w326, y=1) -> (x >= y?=w316:bool)
        n217 = Select(t=0, s=w318, f=3) -> (s? t:f=w317:i32)
        n218 = Select(t=4, s=w316, f=w317) -> (s? t:f=w314:i32)
        n219 = local read "tapeOut"() -> (w319:dbl)
      }
      frame 4 {
        n220 = feedback #11() -> (w334:i8)  [unwired: 1 in]
        n221 = feedback-in #11(w333) -> ()
        n222 = Less?(x=w333, y=w334) -> (x < y?=w332:bool)
        n223 = Select(t=0, s=w332, f=4) -> (s? t:f=w329:i32)
        n224 = global write "Robot Global Data.vi" "finishedRtweak"(TRUE ("finishedRtweak")) -> ()
      }
    }
    n225 = call <vilib>:"WPI_MotorControlSetOutput.vi"("Output"=w218, "MotorControlDevRef"=w227) -> ()  [unwired: 7 in, 3 out]
    n226 = call <vilib>:"WPI_MotorControlSetOutput.vi"("Output"=w225, "MotorControlDevRef"=w226) -> ()  [unwired: 7 in, 3 out]
    n227 = Wait (ms)(milliseconds to wait=u32 20) -> ()  [unwired: 1 out]
  }
  n228 = while {
    shift-right: [w340] -> _
    shift-left: 0 -> [w339]
    tunnel: w23 -> [w337]
    tunnel: w21 -> [w336]
    i -> [w335]
    stop <- FALSE stop-if-true
    n229 = global read "Robot Global Data.vi" "climb num"() -> (w338:i32)
    n230 = case shown="1" w339 {
      tunnel: [w351 w359 w360 w379] -> w340
      tunnel: w338 -> [w350 w359 _ w379]
      tunnel: w337 -> [_ w355 _ _]
      tunnel: w336 -> [w343 w354 _ _]
      tunnel: w335 -> [_ w353 w369 _]
      frame 0, Default {
        n231 = call <vilib>:"WPI_CompressorStart.vi"("CompressorDevRef"=w343) -> ()  [unwired: 9 in, 2 out]
        n232 = Greater Or Equal?(x=w350, y=i8 1) -> (x >= y?=w349:bool)
        n233 = local write "tapeReturnSpeed"(0.0 ("tapeReturnSpeed")) -> ()
        n234 = global write "Robot Global Data.vi" "PTO Engaged"(FALSE ("PTO Engaged")) -> ()
        n235 = global write "Robot Global Data.vi" "PTO speed"(0.0 ("PTO speed")) -> ()
        n236 = Select(t=1, s=w349, f=0) -> (s? t:f=w351:i32)
      }
      frame 1 {
        n237 = call <vilib>:"WPI_CompressorStop.vi"("CompressorDevRef"=w354) -> ()  [unwired: 9 in, 2 out]
        n238 = call <vilib>:"WPI_EncoderReset.vi"("EncoderDevRef"=w355) -> ()  [unwired: 9 in, 2 out]
        n239 = local write "tapeReturnSpeed"(0.0 ("tapeReturnSpeed")) -> ()
        n240 = global write "Robot Global Data.vi" "PTO Engaged"(TRUE ("PTO Engaged")) -> ()
        n241 = global write "Robot Global Data.vi" "PTO speed"(0.0 ("PTO speed")) -> ()
        "timeSaved 3" <- w353
      }
      frame 2 {
        n242 = local read "timeSaved 3"() -> (w370:i32)
        n243 = local read "tapeInPTO"() -> (w362:dbl)
        n244 = global write "Robot Global Data.vi" "PTO Engaged"(TRUE ("PTO Engaged")) -> ()
        n245 = Subtract(x=w369, y=w370) -> (x-y=w371:i32)
        n246 = Absolute Value(x=w362) -> (abs(x)=w364:dbl)
        n247 = Negate(x=w364) -> (-x=w363:dbl)
        n248 = local write "tapeReturnSpeed"(w363) -> ()
        n249 = Greater Or Equal?(x=w371, y="tapeRuntime") -> (x >= y?=w367:bool)
        n250 = Select(t=3, s=w367, f=2) -> (s? t:f=w360:i32)
      }
      frame 3 {
        n251 = Absolute Value(x="tapeInPTO") -> (abs(x)=w375:dbl)
        n252 = Absolute Value(x="PTO speed") -> (abs(x)=w377:dbl)
        n253 = Negate(x=w375) -> (-x=w374:dbl)
        n254 = Negate(x=w377) -> (-x=w376:dbl)
        n255 = local write "tapeReturnSpeed"(w374) -> ()
        n256 = global write "Robot Global Data.vi" "PTO Engaged"(TRUE ("PTO Engaged")) -> ()
        n257 = global write "Robot Global Data.vi" "PTO speed"(w376) -> ()
      }
    }
    n258 = Wait (ms)(milliseconds to wait=u32 20) -> ()  [unwired: 1 out]
  }
  n259 = while {
    shift-right: [w387] -> _
    shift-left: _ -> [w385]
    shift-left: _ -> [w382]
    i -> [w383]
    stop <- FALSE stop-if-true
    n260 = global read "Robot Global Data.vi" "1-Button 8"() -> (w386:bool)
    n261 = case shown="0, Default" w385 {
      tunnel: w386 -> [w397 w434 w453 w479 w506 w528 w550 w563]
      tunnel: [w400 w433 w452 w478 w505 w527 w549 w562] -> w387
      tunnel: w383 -> [_ _ _ _ _ _ _ _]
      tunnel: w382 -> [_ _ w443 w471 w497 w522 w545 _]
      frame 0, Default {
        # "stored var for\nspeedup function"
        # "turnSpeedSlow sets\nturnSpeed7. So\nchange Slow!"
        # "On Rising Edge of Button Press\nMove to Case 1"
        # "reset variables"
        # "not searching"
        n262 = global read "Robot Global Data.vi" "shift state"() -> (w398:bool)
        n263 = And(x=w397, y=w398) -> (x .and. y?=w396:bool)
        n264 = feedback #12() -> (w402:bool)  [unwired: 1 in]
        n265 = feedback-in #12(w396) -> ()
        n266 = global read "Robot Global Data.vi" "CamTargetReal"() -> (w389:dbl)
        n267 = Greater?(x=w396, y=w402) -> (0:w399:bool)
        n268 = local write "turnSpeedStartSlow"("memoryStartAsSlow") -> ()
        n269 = local write "cameraTarget 3"(w389) -> ()
        n270 = local write "turnSpeed 7"("turnSpeedSlow") -> ()
        n271 = Select(t=1, s=w399, f=0) -> (s? t:f=w400:i32)
        n272 = global write "Robot Global Data.vi" "4?"(FALSE ("4?")) -> ()
        n273 = local write "forceLowGear"(FALSE ("forceLowGear")) -> ()
        n274 = local write "aimBot"(0.0 ("aimBot")) -> ()
      }
      frame 1 {
        # "Set Target Angle"
        # "If button released then\nbail-out to case 0."
        n275 = global read "Robot Global Data.vi" "center Y"() -> (w429:dbl)
        n276 = global read "Robot Global Data.vi" "center X"() -> (w425:dbl)
        n277 = expression code="(x/180.0)*pi" "degrees to radians"("viewAngle 3") -> (w412:dbl)
        n278 = Subtract(x=w425, y="cameraTarget 3") -> (x-y=w416:dbl)
        n279 = local read "cameraTarget 3"() -> (w410:dbl)
        n280 = Equal To 0?(x=w429) -> (x = 0?=w427:bool)
        n281 = Equal To 0?(x=w425) -> (x = 0?=w428:bool)
        n282 = global read "Robot Global Data.vi" "center X"() -> (w409:dbl)
        n283 = Tangent(1:w412) -> (0:w418:dbl)
        n284 = Not And(1:w428, 2:w427) -> (0:w426:bool)
        n285 = Multiply(x=w416, y=w418) -> (x*y=w417:dbl)
        n286 = Subtract(x=w409, y=w410) -> (x-y=w408:dbl)
        n287 = Absolute Value(x=w408) -> (abs(x)=w407:dbl)
        n288 = Inverse Tangent(1:w417) -> (0:w415:dbl)
        n289 = Less?(x=w407, y="distToStartAsSlow") -> (x < y?=w405:bool)
        n290 = global write "Robot Global Data.vi" "Camera Target"("cameraTarget 3") -> ()
        n291 = expression code="(x/pi)*180.0" "radians to degrees"(w415) -> (w414:dbl)
        n292 = Select(t=7, s=w405, f=2) -> (s? t:f=w403:i32)
        n293 = feedback #13() -> (w436:bool)  [unwired: 1 in]
        n294 = feedback-in #13(w434) -> ()
        n295 = Select(t=w403, s=w426, f=1) -> (s? t:f=w420:i32)
        n296 = Less?(x=w434, y=w436) -> (x < y?=w435:bool)
        n297 = global read "Robot Global Data.vi" "Yaw"() -> (w430:dbl)
        n298 = Select(t="Angle 2", s=FALSE, f=w414) -> (s? t:f=w423:dbl)
        n299 = Add(x=w423, y=w430) -> (x+y=→"Target Angle 3":dbl)
        n300 = Select(t=0, s=w435, f=w420) -> (s? t:f=w433:i32)
        n301 = local write "forceLowGear"(TRUE ("forceLowGear")) -> ()
      }
      frame 2 {
        # "Build in 2.25 degrees for tire bounce back"
        # "Dont energize motors untill checking\nthreshold against difference."
        # "If button released then\nbail-out to case 0."
        n302 = local read "Target Angle 3"() -> (w449:dbl)
        n303 = global read "Robot Global Data.vi" "Yaw"() -> (w448:dbl)
        n304 = Equal?(x=w443, y=1) -> (x = y?=w441:bool)
        n305 = Subtract(x=w449, y=w448) -> (x-y=w446:dbl)
        n306 = Sign(1:w446) -> (0:w447:dbl)
        n307 = Absolute Value(x=w446) -> (abs(x)=w450:dbl)
        n308 = feedback #14() -> (w455:bool)  [unwired: 1 in]
        n309 = feedback-in #14(w453) -> ()
        n310 = Less?(x=w453, y=w455) -> (x < y?=w454:bool)
        n311 = Less Or Equal?(x=w450, y=15.0 ("aimTolerance")) -> (x <= y?=w451:bool)
        n312 = local read "aimBot"() -> (w440:dbl)
        n313 = Multiply(x=w447, y="turnSpeedHard") -> (x*y=w445:dbl)
        n314 = Select(t=w440, s=w441, f=w445) -> (s? t:f=w444:dbl)
        n315 = local write "aimBot"(w444) -> ()
        n316 = Select(t=3, s=w451, f=2) -> (s? t:f=w457:i32)
        n317 = Select(t=0, s=w454, f=w457) -> (s? t:f=w452:i32)
      }
      frame 3 {
        # "Dont energize motors untill checking\nthreshold against difference."
        # "If button released then\nbail-out to case 0."
        n318 = local read "Target Angle 3"() -> (w476:dbl)
        n319 = global read "Robot Global Data.vi" "Yaw"() -> (w475:dbl)
        n320 = Equal?(x=w471, y=2) -> (x = y?=w469:bool)
        n321 = Subtract(x=w476, y=w475) -> (x-y=w474:dbl)
        n322 = feedback #15() -> (w481:bool)  [unwired: 1 in]
        n323 = feedback-in #15(w479) -> ()
        n324 = local read "aimTolerance 2"() -> (w460:dbl)
        n325 = Absolute Value(x=w474) -> (abs(x)=w477:dbl)
        n326 = Less?(x=w479, y=w481) -> (x < y?=w480:bool)
        n327 = Less Or Equal?(x=w477, y=w460) -> (x <= y?=w465:bool)
        n328 = case shown="True" w465 {
          tunnel: [FALSE w486] -> w462
          frame False {
          }
          frame True {
            n329 = global read "Robot Global Data.vi" "center Y"() -> (w490:dbl)
            n330 = global read "Robot Global Data.vi" "center X"() -> (w487:dbl)
            n331 = Equal To 0?(x=w490) -> (x = 0?=w488:bool)
            n332 = Equal To 0?(x=w487) -> (x = 0?=w489:bool)
            n333 = Not And(1:w489, 2:w488) -> (0:w486:bool)
          }
        }
        n334 = local read "aimBot"() -> (w468:dbl)
        n335 = Sign(1:w474) -> (0:w466:dbl)
        n336 = Multiply(x=w466, y="turnSpeedMedium") -> (x*y=w473:dbl)
        n337 = Select(t=w468, s=w469, f=w473) -> (s? t:f=w472:dbl)
        n338 = local write "aimBot"(w472) -> ()
        n339 = Select(t=6, s=w462, f=4 ("t")) -> (s? t:f=w461:i32)
        n340 = local write "leftOrRight"(w466) -> ()
        n341 = Select(t=w461, s=w465, f=3) -> (s? t:f=w483:i32)
        n342 = Select(t=0, s=w480, f=w483) -> (s? t:f=w478:i32)
      }
      frame 4 {
        # "Dont energize motors untill checking\nthreshold against difference."
        # "If button released then\nbail-out to case 0."
        n343 = local read "Target Angle 3"() -> (w502:dbl)
        n344 = global read "Robot Global Data.vi" "Yaw"() -> (w501:dbl)
        n345 = Equal?(x=w497, y=3) -> (x = y?=w495:bool)
        n346 = Subtract(x=w502, y=w501) -> (x-y=w499:dbl)
        n347 = feedback #16() -> (w508:bool)  [unwired: 1 in]
        n348 = feedback-in #16(w506) -> ()
        n349 = Absolute Value(x=w499) -> (abs(x)=w503:dbl)
        n350 = Less?(x=w506, y=w508) -> (x < y?=w507:bool)
        n351 = Less Or Equal?(x=w503, y=0.5 ("aimTolerance 2")) -> (x <= y?=w504:bool)
        n352 = local read "aimBot"() -> (w494:dbl)
        n353 = Sign(1:w499) -> (0:w500:dbl)
        n354 = Multiply(x=w500, y="turnSpeed 7") -> (x*y=w498:dbl)
        n355 = Select(t=w494, s=w495, f=w498) -> (s? t:f=w491:dbl)
        n356 = Select(t=5, s=w504, f=4) -> (s? t:f=w510:i32)
        n357 = local write "aimBot"(w491) -> ()
        n358 = Select(t=0, s=w507, f=w510) -> (s? t:f=w505:i32)
      }
      frame 6 {
        # "Dont energize motors untill checking\nthreshold against difference."
        # "If button released then\nbail-out to case 0."
        n359 = local read "cameraTarget 3"() -> (w514:dbl)
        n360 = global read "Robot Global Data.vi" "center X"() -> (w515:dbl)
        n361 = Equal?(x=w522, y=3) -> (x = y?=w520:bool)
        n362 = Subtract(x=w515, y=w514) -> (x-y=w524:dbl)
        n363 = Absolute Value(x=w524) -> (abs(x)=w513:dbl)
        n364 = feedback #17() -> (w530:bool)  [unwired: 1 in]
        n365 = feedback-in #17(w528) -> ()
        n366 = local read "turnSpeed 7"() -> (w516:dbl)
        n367 = Less?(x=w528, y=w530) -> (x < y?=w529:bool)
        n368 = local read "aimBot"() -> (w519:dbl)
        n369 = Sign(1:w524) -> (0:w525:dbl)
        n370 = Multiply(x=w525, y=w516) -> (x*y=w523:dbl)
        n371 = Less Or Equal?(x=w513, y=0.01 ("aimTolerance 2")) -> (x <= y?=w526:bool)
        n372 = Select(t=w519, s=w520, f=w523) -> (s? t:f=w517:dbl)
        n373 = Select(t=5, s=w526, f=6) -> (s? t:f=w532:i32)
        n374 = local write "aimBot"(w517) -> ()
        n375 = Select(t=0, s=w529, f=w532) -> (s? t:f=w527:i32)
      }
      frame 7 {
        # "Dont energize motors untill checking\nthreshold against difference."
        # "If button released then\nbail-out to case 0."
        n376 = local read "cameraTarget 3"() -> (w538:dbl)
        n377 = global read "Robot Global Data.vi" "center X"() -> (w539:dbl)
        n378 = Equal?(x=w545, y=3) -> (x = y?=w543:bool)
        n379 = Subtract(x=w539, y=w538) -> (x-y=w547:dbl)
        n380 = Absolute Value(x=w547) -> (abs(x)=w537:dbl)
        n381 = feedback #18() -> (w552:bool)  [unwired: 1 in]
        n382 = feedback-in #18(w550) -> ()
        n383 = Less?(x=w550, y=w552) -> (x < y?=w551:bool)
        n384 = local read "aimBot"() -> (w542:dbl)
        n385 = Sign(1:w547) -> (0:w535:dbl)
        n386 = Multiply(x=w535, y="turnSpeedStartSlow") -> (x*y=w546:dbl)
        n387 = Less Or Equal?(x=w537, y=0.01 ("aimTolerance 2")) -> (x <= y?=w548:bool)
        n388 = Select(t=w542, s=w543, f=w546) -> (s? t:f=w540:dbl)
        n389 = local write "leftOrRight"(w535) -> ()
        n390 = Select(t=5, s=w548, f=7) -> (s? t:f=w554:i32)
        n391 = local write "aimBot"(w540) -> ()
        n392 = Select(t=0, s=w551, f=w554) -> (s? t:f=w549:i32)
      }
      frame 5 {
        # "If button released then\nbail-out to case 0."
        n393 = local read "leftOrRight"() -> (w557:dbl)
        n394 = feedback #19() -> (w565:bool)  [unwired: 1 in]
        n395 = feedback-in #19(w563) -> ()
        n396 = Less?(x=w563, y=w565) -> (x < y?=w564:bool)
        n397 = Multiply(x="holding", y=w557) -> (x*y=w559:dbl)
        n398 = local write "aimBot"(w559) -> ()
        n399 = global write "Robot Global Data.vi" "4?"(TRUE ("4?")) -> ()
        n400 = Select(t=0, s=w564, f=5) -> (s? t:f=w562:i32)
      }
    }
    n401 = global read "Robot Global Data.vi" "4?"() -> (w381:bool)
    n402 = call-poly <vilib>:"NT Write Value.vi"("Boolean"=w381, "Name"="aimed") -> ()  [unwired: 9 in, 1 out]
    n403 = Wait (ms)(milliseconds to wait=u32 20) -> ()  [unwired: 1 out]
    "aimState" <- w385
  }
  n404 = call <vilib>:"WPI_SolenoidRefNum Registry Get.vi"("refnum name"="intakeSol") -> ("error out"=w17:errorcluster, "SolenoidDevRef"=w36:T1)  [unwired: 9 in]
  n405 = call <vilib>:"WPI_MotorControlRefNum Registry Get.vi"("refnum name"="intakeMot") -> ("error out"=w18:errorcluster, "MotorControlDevRef"=w34:T4)  [unwired: 9 in]
  n406 = call <vilib>:"WPI_PotentiometerRefNum Registry Get.vi"("refnum name"="arm pot") -> ("PotDevRef"=w30:T17)  [unwired: 9 in, 1 out]
  n407 = call <vilib>:"WPI_PotentiometerGetNormalized.vi"("PotDevRef"=w30) -> ("Normalized Value"=w29:dbl)  [unwired: 8 in, 2 out]
  n408 = while {
    tunnel: w36 -> [w572]
    tunnel: w34 -> [w580]
    tunnel: w18 -> [w571]
    tunnel: w17 -> [w570]
    stop <- FALSE stop-if-true
    # "Both drivers share\ncontrol of the intake"
    # "Obey in pos (button box). Shot overrides position to\ndown, as does the main driver attempting to intake"
    n409 = global read "Robot Global Data.vi" "in pos override"() -> (w577:bool)
    n410 = global read "Robot Global Data.vi" "in ctl num"() -> (w579:i16)
    n411 = global read "Robot Global Data.vi" "In pos"() -> (w576:bool)
    n412 = global read "Robot Global Data.vi" "1-TopLeft"() -> (w567:bool)
    n413 = Or(x=w577, y=w576) -> (x .or. y?=w569:bool)
    n414 = case shown="1" w579 {
      tunnel: [w589 w593 w594] -> w578
      frame 1 {
        n415 = Negate(x="intake hi") -> (-x=w589:dbl)
      }
      frame 0, Default {
        n416 = global read "Robot Global Data.vi" "1-TopLeft"() -> (w591:bool)
        n417 = local read "intake hi"() -> (w592:dbl)
        n418 = Select(t=w592, s=w591, f=0.0) -> (s? t:f=w593:dbl)
      }
      frame 2 {
        n419 = local read "intake hi"() -> (w594:dbl)
      }
    }
    n420 = Or(x=w569, y=w567) -> (x .or. y?=w568:bool)
    n421 = Select(t=WPI_SolenoidValue."On" ("Value"), s=w568, f=WPI_SolenoidValue."Off" ("Value")) -> (s? t:f=w573:T24)
    n422 = feedback #20() -> (w575:T24)  [unwired: 1 in]
    n423 = feedback-in #20(w573) -> ()
    n424 = Not Equal?(x=w573, y=w575) -> (x != y?=w574:bool)
    n425 = case shown="True" w574 {
      tunnel: w573 -> [_ w587]
      tunnel: w572 -> [_ w586]
      tunnel: w570 -> [_ w585]
      frame False {
      }
      frame True {
        n426 = call-poly <vilib>:"WPI_SolenoidSet.vi"("error in (no error)"=w585, "Value"=w587, "SolenoidDevRef"=w586) -> ()  [unwired: 7 in, 2 out]
      }
    }
    n427 = call <vilib>:"WPI_MotorControlSetOutput.vi"("error in (no error)"=w571, "Output"=w578, "MotorControlDevRef"=w580) -> ()  [unwired: 6 in, 3 out]
    n428 = Wait (ms)(milliseconds to wait=u32 20) -> ()  [unwired: 1 out]
  }
  n429 = while {
    tunnel: w30 -> [w630]
    shift-right: [w629] -> _
    shift-left: w29 -> [w624]
    shift-left: w29 -> [w623]
    shift-left: w29 -> [w622]
    shift-left: w29 -> [w621]
    shift-left: w29 -> [w620]
    shift-left: w29 -> [w619]
    shift-left: w29 -> [w618]
    shift-left: w29 -> [w617]
    shift-left: w29 -> [w616]
    shift-left: w29 -> [w615]
    shift-left: w29 -> [w608]
    shift-left: w29 -> [w607]
    shift-left: w29 -> [w606]
    shift-left: w29 -> [w605]
    shift-left: w29 -> [w604]
    shift-left: w29 -> [w598]
    shift-left: w29 -> [w595]
    stop <- FALSE stop-if-true
    # "This mean-of-medians filtering helped a ton\nwith jumpy potentiometers"
    # "Take last 17 (arbitrary) values, sort them in ascending order\nThrow out the 4 highest and 3 lowest, average the rest"
    n430 = call <vilib>:"WPI_PotentiometerGetNormalized.vi"("PotDevRef"=w630) -> ("Normalized Value"=w629:dbl)  [unwired: 8 in, 2 out]
    n431 = Build Array(w624, w623, w622, w621, w620, w619, w618, w617, w616, w615, w608, w607, w606, w605, w604, w598, w595) -> (w614:dbl[])
    n432 = Sort 1D Array(array=w614) -> (sorted array=w613:dbl[])
    n433 = Index Array(array=w613) -> (element #5=w612:dbl, element #6=w611:dbl, element #7=w610:dbl, element #8=w603:dbl, element #9=w602:dbl, element #10=w601:dbl, element #11=w600:dbl, element #12=w599:dbl, element #13=w597:dbl, element #14=w596:dbl)  [unwired: 17 in, 7 out]
    n434 = Compound Arithmetic op=ADD(w612, w611, w610, w603, w602, w601, w600, w599, w597, w596) -> (w609:dbl)
    n435 = Divide(x=w609, y=10.0) -> (x/y=w627:dbl)
    "arm pot" <- w627
    n436 = global write "Robot Global Data.vi" "arm pot"(w627) -> ()
    n437 = Wait (ms)(milliseconds to wait=u32 10) -> ()  [unwired: 1 out]
  }
  n438 = call <vilib>:"WPI_SolenoidRefNum Registry Get.vi"("refnum name"="low shoot 1") -> ("SolenoidDevRef"=w38:T1)  [unwired: 9 in, 1 out]
  n439 = call <vilib>:"WPI_SolenoidRefNum Registry Get.vi"("refnum name"="low shoot 2") -> ("SolenoidDevRef"=w39:T1)  [unwired: 9 in, 1 out]
  n440 = call <vilib>:"WPI_SolenoidRefNum Registry Get.vi"("refnum name"="high shoot 2") -> ("SolenoidDevRef"=w41:T1)  [unwired: 9 in, 1 out]
  n441 = call <vilib>:"WPI_SolenoidRefNum Registry Get.vi"("refnum name"="high shoot 1") -> ("SolenoidDevRef"=w40:T1)  [unwired: 9 in, 1 out]
  n442 = Bundle("SolenoidDevRef"=w38, "SolenoidDevRef"=w39, "SolenoidDevRef"=w40, "SolenoidDevRef"=w41) -> (w19:T25)  [unwired: 1 in]
  n443 = while {
    tunnel: w19 -> [w638]
    stop <- FALSE stop-if-true
    # "Shot sequence"
    # "Debounce to avoid\ndouble shot"
    n444 = global read "Robot Global Data.vi" "Shoot!"() -> (w633:bool)
    n445 = global read "Robot Global Data.vi" "1-TopCenter"() -> (w632:bool)
    n446 = Or(x=w633, y=w632) -> (x .or. y?=w631:bool)
    n447 = global read "Robot Global Data.vi" "Shot Selector"() -> (w637:bool)
    n448 = feedback #21() -> (w635:bool)  [unwired: 1 in]
    n449 = feedback-in #21(w631) -> ()
    n450 = Greater?(x=w631, y=w635) -> (0:w634:bool)
    n451 = case shown="True" w634 {
      tunnel: w638 -> [_ w647]
      tunnel: w637 -> [_ w646]
      frame False {
        n452 = Wait (ms)(milliseconds to wait=u32 20) -> ()  [unwired: 1 out]
      }
      frame True {
        # "Finish it"
        # "Open up intake"
        n453 = while {
          tunnel: w647 -> [w677]
          tunnel: [w677] -> w645
          tunnel: [w676] -> w642
          stop <- w676 stop-if-true
          w675 = TRUE ("in pos override")
          w676 = TRUE
          n454 = global read "Robot Global Data.vi" "Pins / Intake timing"() -> (w674:dbl)
          n455 = Unbundle(w677) -> ()  [unwired: 4 out]
          n456 = global write "Robot Global Data.vi" "in pos override"(w675) -> ()
          n457 = global write "Robot Global Data.vi" "retainer override"(w675) -> ()
          n458 = Wait (ms)(milliseconds to wait=w674) -> ()  [unwired: 1 out]
        }
        n459 = while {
          tunnel: w646 -> [w663]
          tunnel: w645 -> [w662]
          tunnel: [w661] -> w644
          tunnel: w642 -> [_]
          tunnel: [w660] -> w641
          stop <- w660 stop-if-true
          w660 = TRUE
          # "Shoot!"
          n460 = case shown="False" w663 {
            tunnel: w662 -> [w664 w670]
            tunnel: [w664 w670] -> w661
            frame False {
              w667 = WPI_SolenoidValue."On" ("Value")
              # "Long shot\nFire away!"
              n461 = Unbundle(w664) -> ("SolenoidDevRef"=w669:T1, "SolenoidDevRef"=w668:T1, "SolenoidDevRef"=w666:T1, "SolenoidDevRef"=w665:T1)
              n462 = call-poly <vilib>:"WPI_SolenoidSet.vi"("Value"=w667, "SolenoidDevRef"=w669) -> ()  [unwired: 8 in, 2 out]
              n463 = call-poly <vilib>:"WPI_SolenoidSet.vi"("Value"=w667, "SolenoidDevRef"=w668) -> ()  [unwired: 8 in, 2 out]
              n464 = call-poly <vilib>:"WPI_SolenoidSet.vi"("Value"=w667, "SolenoidDevRef"=w666) -> ()  [unwired: 8 in, 2 out]
              n465 = call-poly <vilib>:"WPI_SolenoidSet.vi"("Value"=w667, "SolenoidDevRef"=w665) -> ()  [unwired: 8 in, 2 out]
            }
            frame True {
              w671 = WPI_SolenoidValue."On" ("Value")
              # "Close shot - low cylinders  only"
              n466 = Unbundle(w670) -> ("SolenoidDevRef"=w673:T1, "SolenoidDevRef"=w672:T1)  [unwired: 2 out]
              n467 = call-poly <vilib>:"WPI_SolenoidSet.vi"("Value"=w671, "SolenoidDevRef"=w673) -> ()  [unwired: 8 in, 2 out]
              n468 = call-poly <vilib>:"WPI_SolenoidSet.vi"("Value"=w671, "SolenoidDevRef"=w672) -> ()  [unwired: 8 in, 2 out]
            }
          }
          n469 = Wait (ms)(milliseconds to wait=u32 350) -> ()  [unwired: 1 out]
        }
        n470 = while {
          tunnel: w644 -> [w653]
          tunnel: [w653] -> w643
          tunnel: w641 -> [_]
          tunnel: [w652] -> w640
          stop <- w652 stop-if-true
          w652 = TRUE
          w656 = WPI_SolenoidValue."Off" ("Value")
          # "Re-cock"
          n471 = Unbundle(w653) -> ("SolenoidDevRef"=w658:T1, "SolenoidDevRef"=w657:T1, "SolenoidDevRef"=w655:T1, "SolenoidDevRef"=w654:T1)
          n472 = Wait (ms)(milliseconds to wait=u32 0) -> ()  [unwired: 1 out]
          n473 = call-poly <vilib>:"WPI_SolenoidSet.vi"("Value"=w656, "SolenoidDevRef"=w658) -> ()  [unwired: 8 in, 2 out]
          n474 = call-poly <vilib>:"WPI_SolenoidSet.vi"("Value"=w656, "SolenoidDevRef"=w657) -> ()  [unwired: 8 in, 2 out]
          n475 = call-poly <vilib>:"WPI_SolenoidSet.vi"("Value"=w656, "SolenoidDevRef"=w655) -> ()  [unwired: 8 in, 2 out]
          n476 = call-poly <vilib>:"WPI_SolenoidSet.vi"("Value"=w656, "SolenoidDevRef"=w654) -> ()  [unwired: 8 in, 2 out]
        }
        n477 = while {
          tunnel: w643 -> [w649]
          tunnel: [w649] -> _
          tunnel: w640 -> [_]
          stop <- TRUE stop-if-true
          w648 = FALSE ("in pos override")
          # "intake and retainer return to\nbutton-box control"
          n478 = Unbundle(w649) -> ()  [unwired: 4 out]
          n479 = global write "Robot Global Data.vi" "in pos override"(w648) -> ()
          n480 = global write "Robot Global Data.vi" "retainer override"(w648) -> ()
        }
      }
    }
  }
  n481 = call <vilib>:"WPI_SolenoidRefNum Registry Get.vi"("refnum name"="retainer") -> ("SolenoidDevRef"=w32:T1)  [unwired: 9 in, 1 out]
  n482 = while {
    stop <- FALSE stop-if-true
    w680 = "popUpCamera" ("refnum name")
    # "Slider on base of joystick activates a \npneumatic popup camera. This switches\ndashboard camera feed, hence sending state\nto dash over NetworkTables"
    n483 = global read "Robot Global Data.vi" "1-slider"() -> (w679:bool)
    n484 = call <vilib>:"WPI_SolenoidRefNum Registry Get.vi"("refnum name"=w680) -> ("SolenoidDevRef"=w684:T1)  [unwired: 9 in, 1 out]
    n485 = Select(t=WPI_SolenoidValue."On", s=w679, f=WPI_SolenoidValue."Off" ("Value")) -> (s? t:f=w683:T24)
    n486 = call-poly <vilib>:"WPI_SolenoidSet.vi"("Value"=w683, "SolenoidDevRef"=w684) -> ()  [unwired: 8 in, 2 out]
    n487 = call-poly <vilib>:"NT Write Value.vi"("Boolean"=w679, "Name"=w680) -> ()  [unwired: 9 in, 1 out]
    n488 = Wait (ms)(milliseconds to wait=u32 20) -> ()  [unwired: 1 out]
  }
  n489 = while {
    tunnel: w32 -> [w692]
    stop <- FALSE stop-if-true
    # "control ball retainer\non = engaged"
    n490 = global read "Robot Global Data.vi" "retainer num"() -> (w688:i16)
    n491 = case shown="2" w688 {
      tunnel: [w696 w697 w704] -> w687
      frame 0, Default {
        w696 = FALSE
        n492 = local write "Retainer Locked On"(w696) -> ()
      }
      frame 1 {
        n493 = global read "Robot Global Data.vi" "retainer override"() -> (w698:bool)
        n494 = Not(x=w698) -> (.not. x?=w697:bool)
      }
      frame 2 {
        # "automatic retainer control.\nIf shooting, disengage it\nIf IR ball sensor thresh crossed, engage it. but prioritize shot (disengage)"
        n495 = global read "Robot Global Data.vi" "ball dist thresh"() -> (w705:dbl)
        n496 = global read "Robot Global Data.vi" "IR dist to ball"() -> (w706:dbl)
        n497 = global read "Robot Global Data.vi" "retainer override"() -> (w703:bool)
        n498 = local write "Retainer Locked On"(FALSE ("Retainer Locked On")) -> ()
        n499 = Greater Or Equal?(x=w706, y=w705) -> (x >= y?=w699:bool)
        n500 = Not(x=w699) -> (.not. x?=w701:bool)
        n501 = Not Or(1:w701, 2:w703) -> (0:w704:bool)
        n502 = call-poly <vilib>:"NT Write Value.vi"("Boolean"=w699, "Name"="haveball") -> ()  [unwired: 9 in, 1 out]
      }
    }
    n503 = Select(t=WPI_SolenoidValue."On" ("Value"), s=w687, f=WPI_SolenoidValue."Off" ("Value")) -> (s? t:f=w690:T24)
    n504 = feedback #22() -> (w693:T24)  [unwired: 1 in]
    n505 = feedback-in #22(w690) -> ()
    n506 = Not Equal?(x=w690, y=w693) -> (x != y?=w694:bool)
    n507 = case shown="True" w694 {
      tunnel: w690 -> [_ w708]
      tunnel: w692 -> [_ w707]
      frame False {
      }
      frame True {
        n508 = call-poly <vilib>:"WPI_SolenoidSet.vi"("Value"=w708, "SolenoidDevRef"=w707) -> ()  [unwired: 8 in, 2 out]
      }
    }
    n509 = Wait (ms)(milliseconds to wait=u32 20) -> ()  [unwired: 1 out]
  }
  n510 = while {
    stop <- FALSE stop-if-true
    w747 = -0.275 ("upper limit")
    w749 = -0.8 ("upper limit")
    w754 = 0.275 ("upper limit")
    w742 = 0.8 ("upper limit")
    # "Force range on arm"
    # "This is where we apply a fudge\nfactor to the arm's position\nto be used when another function\ncontrols the arms. This is auto\ncheval sequence as well as stowing\narms during the climb"
    # "significant deadband on\ninput, so this gives\nfaily even \"true\" ranges"
    # "2-stage bang-bang position control"
    # "DIO jumper on practice bot tells me which I'm running, avoids mechanism destroying itself from bad limit"
    # "Segment button box potentiometer into 5 ranges"
    # "Arm PID on Pot Ranges"
    n511 = global read "Robot Global Data.vi" "Arm Control"() -> (w741:dbl)
    n512 = In Range and Coerce(upper limit=w747, x=w741, lower limit=w749) -> (In Range?=w752:bool)  [unwired: 1 out]
    n513 = In Range and Coerce(upper limit=w742, x=w741, lower limit=w754) -> (In Range?=w763:bool)  [unwired: 1 out]
    n514 = In Range and Coerce(upper limit=w754, x=w741, lower limit=w747) -> (In Range?=w762:bool)  [unwired: 1 out]
    n515 = In Range and Coerce(upper limit=w749, x=w741, lower limit=-1.0) -> (In Range?=w761:bool)  [unwired: 1 out]
    n516 = In Range and Coerce(upper limit=1.001, x=w741, lower limit=w742) -> (In Range?=w746:bool)  [unwired: 1 out]
    n517 = Select(t=i8 4, s=w752, f=i8 0) -> (s? t:f=w748:i8)
    n518 = Select(t=i8 2, s=w763, f=i8 0) -> (s? t:f=w764:i8)
    n519 = Select(t=i8 5, s=w761, f=i8 0) -> (s? t:f=w753:i8)
    n520 = Select(t=i8 1, s=w746, f=i8 0) -> (s? t:f=w740:i8)
    n521 = Select(t=i8 3, s=w762, f=i8 0) -> (s? t:f=w765:i8)
    n522 = Compound Arithmetic op=ADD(w740, w764, w765, w748, w753) -> (w738:i8)
    n523 = global read "Robot Global Data.vi" "arm override"() -> (w724:bool)
    n524 = case shown="False" w724 {
      tunnel: w738 -> [w766 _]
      tunnel: [w767 w781] -> w720
      frame False {
        # "Various arm setpoints"
        n525 = global read "Robot Global Data.vi" "arm extended"() -> (w768:dbl)
        n526 = case shown="4" w766 {
          tunnel: w768 -> [_ w770 w775 w778 w779]
          tunnel: [w769 w771 w773 w776 w779] -> w767
          frame 1, Default {
            # "Start"
            n527 = global read "Robot Global Data.vi" "arm stow"() -> (w769:dbl)
          }
          frame 2 {
            # "Vertical"
            n528 = Add(x=w770, y="arm vert offset") -> (x+y=w771:dbl)
          }
          frame 3 {
            # "Cheval"
            n529 = Add(x=w775, y="arm cdf offset") -> (x+y=w773:dbl)
          }
          frame 4 {
            # "Straight extended"
            n530 = Add(x=w778, y="arm horiz offset") -> (x+y=w776:dbl)
          }
          frame 5 {
            # "Porticullis"
          }
        }
      }
      frame True {
        # "1:1 control between driver\ninterface and arm position\nRarely used but helpful\nfeature, occasionally"
        # "Force input of [-1, 1] to scale\n exactly to [min, max]"
        n531 = global read "Robot Global Data.vi" "arm stow"() -> (w786:dbl)
        n532 = global read "Robot Global Data.vi" "arm extended"() -> (w789:dbl)
        n533 = global read "Robot Global Data.vi" "Arm Control"() -> (w780:dbl)
        n534 = Subtract(x=w786, y=w789) -> (x-y=w790:dbl)
        n535 = Absolute Value(x=w790) -> (abs(x)=w783:dbl)
        n536 = Compound Arithmetic op=MULTIPLY(w780, w783, 0.5 ("value")) -> (w787:dbl)
        n537 = Add(x=w787, y=w786) -> (x+y=w785:dbl)
        n538 = Divide(x=w783, y=2.0) -> (x/y=w784:dbl)
        n539 = Subtract(x=w785, y=w784) -> (x-y=w781:dbl)
      }
    }
    n540 = global read "Robot Global Data.vi" "tapesModArm"() -> (w709:bool)
    n541 = Add(x="modifyArm", y=w720) -> (x+y=w714:dbl)
    n542 = Select(t=1.0, s=w709, f=0.0) -> (s? t:f=w712:dbl)
    n543 = Add(x=w714, y=w712) -> (x+y=w713:dbl)
    n544 = global read "Robot Global Data.vi" "IsPracticeBot?"() -> (w715:bool)
    n545 = global read "Robot Global Data.vi" "arm extended"() -> (w726:dbl)
    n546 = global read "Robot Global Data.vi" "arm stow"() -> (w725:dbl)
    n547 = In Range and Coerce(upper limit=w725, x=w713, lower limit=w726) -> (coerced(x)=w723:dbl)  [unwired: 1 out]
    n548 = Select(t="practiceOffset", s=w715, f=0.0) -> (s? t:f=w717:dbl)
    n549 = Add(x=w717, y=w723) -> (x+y=w722:dbl)
    n550 = global read "Robot Global Data.vi" "arm slow spot"() -> (w730:dbl)
    n551 = global read "Robot Global Data.vi" "arm speed slow"() -> (w728:dbl)
    n552 = global read "Robot Global Data.vi" "arm pot"() -> (w732:dbl)
    n553 = global read "Robot Global Data.vi" "arm speed"() -> (w729:dbl)
    n554 = call "Bang-bang.vi"("Feedback"=w732, "Target"=w722, "Tolerance"=0.015, "Slow point"=w730, "Low Speed"=w728, "High Speed"=w729) -> ("Out speed"=w727:dbl)
    n555 = Negate(x=w727) -> (-x=w721:dbl)
    "arm output" <- w721
    n556 = call <vilib>:"WPI_MotorControlRefNum Registry Get.vi"("refnum name"="arm motor") -> ("error out"=w736:errorcluster, "MotorControlDevRef"=w735:T4)  [unwired: 9 in]
    n557 = Wait (ms)(milliseconds to wait=u32 20) -> ()  [unwired: 1 out]
    n558 = call <vilib>:"WPI_MotorControlSetOutput.vi"("error in (no error)"=w736, "Output"=w721, "MotorControlDevRef"=w735) -> ()  [unwired: 6 in, 3 out]
    n559 = global write "Robot Global Data.vi" "arm out"(w721) -> ()
  }
  n560 = while {
    shift-right: [w794] -> _
    shift-left: _ -> [w792]
    stop <- FALSE stop-if-true
    # "What this does, at a glance:\nCase 0: \"Normal case\"\n1: Drive forward slowly until IR sensor\nsees cheval for 3 cycles\n2: Drive a specified encoder distance\n(varied between 0 to 3 inches)\n3: Lower the arms as far as possible, at\na greater speed than the normal maximum.\nContinue for specified distance (2 feet)\n4: Release control of arms to driver,\nincrease speed. Reset arm speed.\n5: Hold y-override until button is released"
    # "Automatic Cheval de Frise crossing sequence. Executes while driver holds\na button and runs until button is let go or sequence is completed. Takes control of\njoystick y- but not x-axis, allowing the driver to steer during the sequence"
    n561 = global read "Robot Global Data.vi" "1-Button 5"() -> (w793:bool)
    n562 = case shown="2" w792 {
      tunnel: w793 -> [w802 w819 w835 w849 w865 w871]
      tunnel: [w806 w818 w831 w845 w864 w870] -> w794
      frame 0, Default {
        # "On Rising Edge of Button Press\nMove to Case 1 if Arm in Cheval Seek Position"
        # "reset variables"
        # "not searching"
        n563 = global read "Robot Global Data.vi" "arm speed normal"() -> (w798:dbl)
        n564 = global read "Robot Global Data.vi" "arm slow spot normal"() -> (w797:dbl)
        n565 = global read "Robot Global Data.vi" "shift state"() -> (w800:bool)
        n566 = And(x=w802, y=w800) -> (x .and. y?=w801:bool)
        n567 = global write "Robot Global Data.vi" "arm speed"(w798) -> ()
        n568 = global write "Robot Global Data.vi" "arm slow spot"(w797) -> ()
        n569 = feedback #23() -> (w809:bool)  [unwired: 1 in]
        n570 = feedback-in #23(w801) -> ()
        n571 = Greater?(x=w801, y=w809) -> (0:w796:bool)
        n572 = Select(t=1, s=w796, f=0) -> (s? t:f=w806:i32)
        n573 = local write "y-override speed"(-0.6 ("speedBot")) -> ()
        n574 = local write "Y-overide"(FALSE ("Y-overide")) -> ()
        n575 = local write "forceLowGear"(FALSE) -> ()
        n576 = local write "modifyArm"(0.0 ("modifyArm")) -> ()
      }
      frame 1 {
        # "If IR detects the high edge of the CDF 3 consecutive loop cycles \nthen record current encoder setting and proceed to Case 2."
        # "If button released then\nbail-out to case 0."
        n577 = global read "Robot Global Data.vi" "IR dist to CDF"() -> (w827:dbl)
        n578 = Greater Or Equal?(x=w827, y=0.4) -> (x >= y?=w815:bool)
        n579 = feedback-in #24(w815) -> ()
        n580 = feedback #24() -> (w814:bool)  [unwired: 1 in]
        n581 = feedback #25() -> (w813:bool)  [unwired: 1 in]
        n582 = feedback-in #25(w814) -> ()
        n583 = Compound Arithmetic op=AND(w815, w814, w813) -> (w812:bool)
        n584 = feedback #26() -> (w821:bool)  [unwired: 1 in]
        n585 = feedback-in #26(w819) -> ()
        n586 = Less?(x=w819, y=w821) -> (x < y?=w820:bool)
        n587 = Select(t=2, s=w812, f=1) -> (s? t:f=w823:i32)
        n588 = Select(t=0, s=w820, f=w823) -> (s? t:f=w818:i32)
        n589 = local write "Y-overide"(TRUE ("Y-overide")) -> ()
        n590 = local write "forceLowGear"(TRUE) -> ()
        n591 = global read "Robot Global Data.vi" "Distance (enc.)"() -> (→"rememberEnc":dbl)
        n592 = local write "modifyArm"(0.0 ("modifyArm")) -> ()
      }
      frame 2 {
        # "If button released then\nbail-out to case 0."
        # "Wait for encoder to increase by \"distToLower\"\nthen proceed to Case 3."
        n593 = global read "Robot Global Data.vi" "Distance (enc.)"() -> (w830:dbl)
        n594 = local read "rememberEnc"() -> (w832:dbl)
        n595 = global read "Robot Global Data.vi" "arm slow spot cdf"() -> (w828:dbl)
        n596 = Add(x=w832, y="distToLower") -> (x+y=w833:dbl)
        n597 = global read "Robot Global Data.vi" "arm speed shovel"() -> (w829:dbl)
        n598 = Greater Or Equal?(x=w830, y=w833) -> (x >= y?=w842:bool)
        n599 = feedback #27() -> (w837:bool)  [unwired: 1 in]
        n600 = feedback-in #27(w835) -> ()
        n601 = Less?(x=w835, y=w837) -> (x < y?=w836:bool)
        n602 = global write "Robot Global Data.vi" "arm slow spot"(w828) -> ()
        n603 = Select(t=3, s=w842, f=2) -> (s? t:f=w839:i32)
        n604 = global write "Robot Global Data.vi" "arm speed"(w829) -> ()
        n605 = Select(t=0, s=w836, f=w839) -> (s? t:f=w831:i32)
      }
      frame 3 {
        # "If button released then\nbail-out to case 0."
        # "Wait for encoder to increase by \"distToRaise\"\nthen proceed to Case 4."
        n606 = global read "Robot Global Data.vi" "Distance (enc.)"() -> (w844:dbl)
        n607 = local read "rememberEnc"() -> (w846:dbl)
        n608 = Add(x=w846, y="distToRaise") -> (x+y=w847:dbl)
        n609 = Greater Or Equal?(x=w844, y=w847) -> (x >= y?=w856:bool)
        n610 = local write "modifyArm"(-1.0 ("modifyArm")) -> ()
        n611 = feedback #28() -> (w851:bool)  [unwired: 1 in]
        n612 = feedback-in #28(w849) -> ()
        n613 = Less?(x=w849, y=w851) -> (x < y?=w850:bool)
        n614 = Select(t=4, s=w856, f=3) -> (s? t:f=w853:i32)
        n615 = Select(t=0, s=w850, f=w853) -> (s? t:f=w845:i32)
      }
      frame 4 {
        # "If button released then\nbail-out to case 0."
        # "Move arm back to start and immediately go on to case 5"
        n616 = local read "arm cdf offset"() -> (w861:dbl)
        n617 = global read "Robot Global Data.vi" "arm stow"() -> (w862:dbl)
        n618 = global read "Robot Global Data.vi" "arm slow spot normal"() -> (w857:dbl)
        n619 = global read "Robot Global Data.vi" "arm speed normal"() -> (w858:dbl)
        n620 = Subtract(x=w862, y=w861) -> (x-y=w860:dbl)
        n621 = local write "modifyArm"(w860) -> ()
        n622 = global write "Robot Global Data.vi" "arm slow spot"(w857) -> ()
        n623 = global write "Robot Global Data.vi" "arm speed"(w858) -> ()
        n624 = feedback #29() -> (w867:bool)  [unwired: 1 in]
        n625 = feedback-in #29(w865) -> ()
        n626 = Less?(x=w865, y=w867) -> (x < y?=w866:bool)
        n627 = Select(t=0, s=w866, f=5 ("t")) -> (s? t:f=w864:i32)
        n628 = local write "y-override speed"(-0.8 ("speedBot")) -> ()
      }
      frame 5 {
        # "If button released then\nbail-out to case 0."
        n629 = feedback #30() -> (w873:bool)  [unwired: 1 in]
        n630 = feedback-in #30(w871) -> ()
        n631 = Less?(x=w871, y=w873) -> (x < y?=w872:bool)
        n632 = Select(t=0, s=w872, f=5 ("t")) -> (s? t:f=w870:i32)
      }
    }
    n633 = Wait (ms)(milliseconds to wait=u32 20) -> ()  [unwired: 1 out]
  }
